vi "Text control 2 v4.7_pump-specific.vi"() -> ()   [LabVIEW 2016]
panel:
  in  "Tab Control":enum32{"Main", "Other parameters"}(tab)
  out "Line running":i32
  out "Total lines":i32
  out "Path":path=path "C:/users/rlp38/09Apr2009LTtesting/test2.txt"
  out "I vs Vg":cluster{"Y data in":dbl[], "X data in":dbl[]}[](graph)
  out "Is":dbl format="%.2e"
  out "Id":dbl format="%.2e"
  out "Ig":dbl format="%.2e"
  out "Id max vs time":cluster{"Y data in":dbl[], "X data in":dbl[]}[](graph)
  out "Id min vs time":cluster{"Y data in":dbl[], "X data in":dbl[]}[](graph)
  out "I vs Vd":cluster{"Y data in":dbl[], "X data in":dbl[]}[](graph)
  in  "Program":string="# Set time units to minutes.\n# Change filenames\n#-------------------------------------------------------\n# Port settings\n# Port 1: Nothing\n# Port 2: To sample\n# Port 3: Ultrapure water\n# Port 4: Nothing\n# Port 5: Nothing\n# Port 6: Nothing\n#-------------------------------------------------------\n# Execution time: 8 x 30 = 240 minutes = 4 hours\n# This script is designed to perform a cycling experiment between two liquids.\n# There are 8 pumping cycles, each one followed by 30 minutes of measurements.\n# All cycles pump ultrapure water (port 3).\n# Flow V = 20 pulses/second (400 ul/min)\n#-------------------------------------------------------\n# Cycle 1\npump /1ZR #initialize pump\npump /1Q #query pump\nwait-min 1 #wait 1 minute\npump /1N0R #set step resolution: 0.01 mm\npump /1Q #query pump\nwait 1000 #wait 1 second\npump /1V300R #choose speed: 300 steps/s\npump /1Q #query pump\nwait 1000 #wait 1 second\npump /1O3R #go to port 3, counterclockwise rotation\npump /1Q #query pump\nwait 1000 #wait 1 second\npump /1A2400R #go to absolute position 2400\nwait 20000 #wait 20 seconds\npump /1V20R #set speed to 20 steps/s\npump /1Q #query pump\nwait 10000 # wait 10 seconds\npump /1O2R #switch to port 2, counterclockwise rotation\npump /1Q #query pump\nwait 200 #wait 200 milliseconds\npump /1A0R #go to absolute position 0 (= empty syringe)\ntransfer d 1 -1 -0.1 -1 -1 0\npump /1Q #query pump\ntransfer d 1 -1 -0.1 -1 -1 0\npump /1? #report absolute plunger position\ntransfer d 1 -1 -0.1 -1 -1 0\nwait-min 1\npump /1Q #query pump\npump /1? #report absolute plunger position\ntransfer d 1 -1 -0.1 -1 -1 0\nwait-min 1\npump /1Q #query pump\npump /1? #report absolute plunger position\ntransfer d 1 -1 -0.1 -1 -1 0\nwait-min 1\npump /1Q #query pump\npump /1? #report absolute plunger position\ntransfer d 1 -1 -0.1 -1 -1 0\nwait-min 1\npump /1Q #query pump\npump /1? #report absolute plunger position\ntransfer d 1 -1 -0.1 -1 -1 0\nwait-min 1\npump /1Q #query pump\npump /1? #report absolute plunger position\ntransfer d 1 -1 -0.1 -1 -1 0\nwait-min 1\npump /1Q #query pump\npump /1? #report absolute plunger position\ntransfer d 1 -1 -0.1 -1 -1 0\nwait-min 1\npump /1Q #query pump\npump /1? #report absolute plunger position\ntransfer d 1 -1 -0.1 -1 -1 0\nwait-min 1\npump /1Q #query pump\npump /1? #report absolute plunger position\ntransfer d 1 -1 -0.1 -1 -1 0\nwait-min 1\npump /1Q #query pump\npump /1? #report absolute plunger position\ntransfer d 1 -1 -0.1 -1 -1 0\nwait-min 1\npump /1Q #query pump\npump /1? #report absolute plunger position\ntransfer d 1 -1 -0.1 -1 -1 0\nwait-min 1\npump /1Q #query pump\npump /1? #report absolute plunger position\ntransfer d 1 -1 -0.1 -1 -1 0\nwait-min 1\npump /1Q #query pump\npump /1? #report absolute plunger position\ntransfer d 1 -1 -0.1 -1 -1 0\nwait-min 1\npump /1Q #query pump\npump /1? #report absolute plunger position\ntransfer d 1 -1 -0.1 -1 -1 0\nwait-min 1\npump /1Q #query pump\npump /1? #report absolute plunger position\ntransfer d 1 -1 -0.1 -1 -1 0\nwait-min 1\npump /1Q #query pump\npump /1? #report absolute plunger position\ntransfer d 1 -1 -0.1 -1 -1 0\nwait-min 1\npump /1Q #query pump\npump /1? #report absolute plunger position\ntransfer d 1 -1 -0.1 -1 -1 0\nwait-min 1\npump /1Q #query pump\npump /1? #report absolute plunger position\ntransfer d 1 -1 -0.1 -1 -1 0\nwait-min 1\npump /1Q #query pump\npump /1? #report absolute plunger position\ntransfer d 1 -1 -0.1 -1 -1 0\nwait-min 1\npump /1Q #query pump\npump /1? #report absolute plunger position\ntransfer d 1 -1 -0.1 -1 -1 0\nwait-min 1\npump /1Q #query pump\npump /1? #report absolute plunger position\ntransfer d 1 -1 -0.1 -1 -1 0\nwait-min 1\npump /1Q #query pump\npump /1? #report absolute plunger position\ntransfer d 1 -1 -0.1 -1 -1 0\nwait-min 1\npump /1Q #query pump\npump /1? #report absolute plunger position\ntransfer d 1 -1 -0.1 -1 -1 0\nwait-min 1\npump /1Q #query pump\npump /1? #report absolute plunger position\ntransfer d 1 -1 -0.1 -1 -1 0\nwait-min 1\npump /1Q #query pump\npump /1? #report absolute plunger position\ntransfer d 1 -1 -0.1 -1 -1 0\nwait-min 1\n#-------------------------------------------------------\n# Cycle 2\npump /1ZR #initialize pump\npump /1Q #query pump\nwait-min 1 #wait 1 minute\npump /1N0R #set step resolution: 0.01 mm\npump /1Q #query pump\nwait 1000 #wait 1 second\npump /1V300R #choose speed: 300 steps/s\npump /1Q #query pump\nwait 1000 #wait 1 second\npump /1O3R #go to port 3, counterclockwise rotation\npump /1Q #query pump\nwait 1000 #wait 1 second\npump /1A2400R #go to absolute position 2400\nwait 30000 #wait 30 seconds \npump /1V20R #set speed to 20 steps/s\npump /1Q #query pump\nwait 10000 # wait 10 seconds\npump /1O2R #switch to port 2, counterclockwise rotation\npump /1Q #query pump\nwait 200 #wait 200 milliseconds\npump /1A0R #go to absolute position 0 (= empty syringe)\ntransfer d 1 -1 -0.1 -1 -1 0\npump /1Q #query pump\ntransfer d 1 -1 -0.1 -1 -1 0\npump /1? #report absolute plunger position\ntransfer d 1 -1 -0.1 -1 -1 0\nwait-min 1\npump /1Q #query pump\npump /1? #report absolute plunger position\ntransfer d 1 -1 -0.1 -1 -1 0\nwait-min 1\npump /1Q #query pump\npump /1? #report absolute plunger position\ntransfer d 1 -1 -0.1 -1 -1 0\nwait-min 1\npump /1Q #query pump\npump /1? #report absolute plunger position\ntransfer d 1 -1 -0.1 -1 -1 0\nwait-min 1\npump /1Q #query pump\npump /1? #report absolute plunger position\ntransfer d 1 -1 -0.1 -1 -1 0\nwait-min 1\npump /1Q #query pump\npump /1? #report absolute plunger position\ntransfer d 1 -1 -0.1 -1 -1 0\nwait-min 1\npump /1Q #query pump\npump /1? #report absolute plunger position\ntransfer d 1 -1 -0.1 -1 -1 0\nwait-min 1\npump /1Q #query pump\npump /1? #report absolute plunger position\ntransfer d 1 -1 -0.1 -1 -1 0\nwait-min 1\npump /1Q #query pump\npump /1? #report absolute plunger position\ntransfer d 1 -1 -0.1 -1 -1 0\nwait-min 1\npump /1Q #query pump\npump /1? #report absolute plunger position\ntransfer d 1 -1 -0.1 -1 -1 0\nwait-min 1\npump /1Q #query pump\npump /1? #report absolute plunger position\ntransfer d 1 -1 -0.1 -1 -1 0\nwait-min 1\npump /1Q #query pump\npump /1? #report absolute plunger position\ntransfer d 1 -1 -0.1 -1 -1 0\nwait-min 1\npump /1Q #query pump\npump /1? #report absolute plunger position\ntransfer d 1 -1 -0.1 -1 -1 0\nwait-min 1\npump /1Q #query pump\npump /1? #report absolute plunger position\ntransfer d 1 -1 -0.1 -1 -1 0\nwait-min 1\npump /1Q #query pump\npump /1? #report absolute plunger position\ntransfer d 1 -1 -0.1 -1 -1 0\nwait-min 1\npump /1Q #query pump\npump /1? #report absolute plunger position\ntransfer d 1 -1 -0.1 -1 -1 0\nwait-min 1\npump /1Q #query pump\npump /1? #report absolute plunger position\ntransfer d 1 -1 -0.1 -1 -1 0\nwait-min 1\npump /1Q #query pump\npump /1? #report absolute plunger position\ntransfer d 1 -1 -0.1 -1 -1 0\nwait-min 1\npump /1Q #query pump\npump /1? #report absolute plunger position\ntransfer d 1 -1 -0.1 -1 -1 0\nwait-min 1\npump /1Q #query pump\npump /1? #report absolute plunger position\ntransfer d 1 -1 -0.1 -1 -1 0\nwait-min 1\npump /1Q #query pump\npump /1? #report absolute plunger position\ntransfer d 1 -1 -0.1 -1 -1 0\nwait-min 1\npump /1Q #query pump\npump /1? #report absolute plunger position\ntransfer d 1 -1 -0.1 -1 -1 0\nwait-min 1\npump /1Q #query pump\npump /1? #report absolute plunger position\ntransfer d 1 -1 -0.1 -1 -1 0\nwait-min 1\npump /1Q #query pump\npump /1? #report absolute plunger position\ntransfer d 1 -1 -0.1 -1 -1 0\nwait-min 1\npump /1Q #query pump\npump /1? #report absolute plunger position\ntransfer d 1 -1 -0.1 -1 -1 0\nwait-min 1\n#-------------------------------------------------------\n# Cycle 3\npump /1ZR #initialize pump\npump /1Q #query pump\nwait-min 1 #wait 1 minute\npump /1N0R #set step resolution: 0.01 mm\npump /1Q #query pump\nwait 1000 #wait 1 second\npump /1V300R #choose speed: 300 steps/s\npump /1Q #query pump\nwait 1000 #wait 1 second\npump /1O3R #go to port 3, counterclockwise rotation\npump /1Q #query pump\nwait 1000 #wait 1 second\npump /1A2400R #go to absolute position 2400\nwait 30000 #wait 30 seconds \npump /1V20R #set speed to 20 steps/s\npump /1Q #query pump\nwait 10000 # wait 10 seconds\npump /1O2R #switch to port 2, counterclockwise rotation\npump /1Q #query pump\nwait 200 #wait 200 milliseconds\npump /1A0R #go to absolute position 0 (= empty syringe)\ntransfer d 1 -1 -0.1 -1 -1 0\npump /1Q #query pump\ntransfer d 1 -1 -0.1 -1 -1 0\npump /1? #report absolute plunger position\ntransfer d 1 -1 -0.1 -1 -1 0\nwait-min 1\npump /1Q #query pump\npump /1? #report absolute plunger position\ntransfer d 1 -1 -0.1 -1 -1 0\nwait-min 1\npump /1Q #query pump\npump /1? #report absolute plunger position\ntransfer d 1 -1 -0.1 -1 -1 0\nwait-min 1\npump /1Q #query pump\npump /1? #report absolute plunger position\ntransfer d 1 -1 -0.1 -1 -1 0\nwait-min 1\npump /1Q #query pump\npump /1? #report absolute plunger position\ntransfer d 1 -1 -0.1 -1 -1 0\nwait-min 1\npump /1Q #query pump\npump /1? #report absolute plunger position\ntransfer d 1 -1 -0.1 -1 -1 0\nwait-min 1\npump /1Q #query pump\npump /1? #report absolute plunger position\ntransfer d 1 -1 -0.1 -1 -1 0\nwait-min 1\npump /1Q #query pump\npump /1? #report absolute plunger position\ntransfer d 1 -1 -0.1 -1 -1 0\nwait-min 1\npump /1Q #query pump\npump /1? #report absolute plunger position\ntransfer d 1 -1 -0.1 -1 -1 0\nwait-min 1\npump /1Q #query pump\npump /1? #report absolute plunger position\ntransfer d 1 -1 -0.1 -1 -1 0\nwait-min 1\npump /1Q #query pump\npump /1? #report absolute plunger position\ntransfer d 1 -1 -0.1 -1 -1 0\nwait-min 1\npump /1Q #query pump\npump /1? #report absolute plunger position\ntransfer d 1 -1 -0.1 -1 -1 0\nwait-min 1\npump /1Q #query pump\npump /1? #report absolute plunger position\ntransfer d 1 -1 -0.1 -1 -1 0\nwait-min 1\npump /1Q #query pump\npump /1? #report absolute plunger position\ntransfer d 1 -1 -0.1 -1 -1 0\nwait-min 1\npump /1Q #query pump\npump /1? #report absolute plunger position\ntransfer d 1 -1 -0.1 -1 -1 0\nwait-min 1\npump /1Q #query pump\npump /1? #report absolute plunger position\ntransfer d 1 -1 -0.1 -1 -1 0\nwait-min 1\npump /1Q #query pump\npump /1? #report absolute plunger position\ntransfer d 1 -1 -0.1 -1 -1 0\nwait-min 1\npump /1Q #query pump\npump /1? #report absolute plunger position\ntransfer d 1 -1 -0.1 -1 -1 0\nwait-min 1\npump /1Q #query pump\npump /1? #report absolute plunger position\ntransfer d 1 -1 -0.1 -1 -1 0\nwait-min 1\npump /1Q #query pump\npump /1? #report absolute plunger position\ntransfer d 1 -1 -0.1 -1 -1 0\nwait-min 1\npump /1Q #query pump\npump /1? #report absolute plunger position\ntransfer d 1 -1 -0.1 -1 -1 0\nwait-min 1\npump /1Q #query pump\npump /1? #report absolute plunger position\ntransfer d 1 -1 -0.1 -1 -1 0\nwait-min 1\npump /1Q #query pump\npump /1? #report absolute plunger position\ntransfer d 1 -1 -0.1 -1 -1 0\nwait-min 1\npump /1Q #query pump\npump /1? #report absolute plunger position\ntransfer d 1 -1 -0.1 -1 -1 0\nwait-min 1\npump /1Q #query pump\npump /1? #report absolute plunger position\ntransfer d 1 -1 -0.1 -1 -1 0\nwait-min 1\n#-------------------------------------------------------\n# Cycle 4\npump /1ZR #initialize pump\npump /1Q #query pump\nwait-min 1 #wait 1 minute\npump /1N0R #set step resolution: 0.01 mm\npump /1Q #query pump\nwait 1000 #wait 1 second\npump /1V300R #choose speed: 300 steps/s\npump /1Q #query pump\nwait 1000 #wait 1 second\npump /1O3R #go to port 3, counterclockwise rotation\npump /1Q #query pump\nwait 1000 #wait 1 second\npump /1A2400R #go to absolute position 2400\nwait 30000 #wait 30 seconds \npump /1V20R #set speed to 20 steps/s\npump /1Q #query pump\nwait 10000 # wait 10 seconds\npump /1O2R #switch to port 2, counterclockwise rotation\npump /1Q #query pump\nwait 200 #wait 200 milliseconds\npump /1A0R #go to absolute position 0 (= empty syringe)\ntransfer d 1 -1 -0.1 -1 -1 0\npump /1Q #query pump\ntransfer d 1 -1 -0.1 -1 -1 0\npump /1? #report absolute plunger position\ntransfer d 1 -1 -0.1 -1 -1 0\nwait-min 1\npump /1Q #query pump\npump /1? #report absolute plunger position\ntransfer d 1 -1 -0.1 -1 -1 0\nwait-min 1\npump /1Q #query pump\npump /1? #report absolute plunger position\ntransfer d 1 -1 -0.1 -1 -1 0\nwait-min 1\npump /1Q #query pump\npump /1? #report absolute plunger position\ntransfer d 1 -1 -0.1 -1 -1 0\nwait-min 1\npump /1Q #query pump\npump /1? #report absolute plunger position\ntransfer d 1 -1 -0.1 -1 -1 0\nwait-min 1\npump /1Q #query pump\npump /1? #report absolute plunger position\ntransfer d 1 -1 -0.1 -1 -1 0\nwait-min 1\npump /1Q #query pump\npump /1? #report absolute plunger position\ntransfer d 1 -1 -0.1 -1 -1 0\nwait-min 1\npump /1Q #query pump\npump /1? #report absolute plunger position\ntransfer d 1 -1 -0.1 -1 -1 0\nwait-min 1\npump /1Q #query pump\npump /1? #report absolute plunger position\ntransfer d 1 -1 -0.1 -1 -1 0\nwait-min 1\npump /1Q #query pump\npump /1? #report absolute plunger position\ntransfer d 1 -1 -0.1 -1 -1 0\nwait-min 1\npump /1Q #query pump\npump /1? #report absolute plunger position\ntransfer d 1 -1 -0.1 -1 -1 0\nwait-min 1\npump /1Q #query pump\npump /1? #report absolute plunger position\ntransfer d 1 -1 -0.1 -1 -1 0\nwait-min 1\npump /1Q #query pump\npump /1? #report absolute plunger position\ntransfer d 1 -1 -0.1 -1 -1 0\nwait-min 1\npump /1Q #query pump\npump /1? #report absolute plunger position\ntransfer d 1 -1 -0.1 -1 -1 0\nwait-min 1\npump /1Q #query pump\npump /1? #report absolute plunger position\ntransfer d 1 -1 -0.1 -1 -1 0\nwait-min 1\npump /1Q #query pump\npump /1? #report absolute plunger position\ntransfer d 1 -1 -0.1 -1 -1 0\nwait-min 1\npump /1Q #query pump\npump /1? #report absolute plunger position\ntransfer d 1 -1 -0.1 -1 -1 0\nwait-min 1\npump /1Q #query pump\npump /1? #report absolute plunger position\ntransfer d 1 -1 -0.1 -1 -1 0\nwait-min 1\npump /1Q #query pump\npump /1? #report absolute plunger position\ntransfer d 1 -1 -0.1 -1 -1 0\nwait-min 1\npump /1Q #query pump\npump /1? #report absolute plunger position\ntransfer d 1 -1 -0.1 -1 -1 0\nwait-min 1\npump /1Q #query pump\npump /1? #report absolute plunger position\ntransfer d 1 -1 -0.1 -1 -1 0\nwait-min 1\npump /1Q #query pump\npump /1? #report absolute plunger position\ntransfer d 1 -1 -0.1 -1 -1 0\nwait-min 1\npump /1Q #query pump\npump /1? #report absolute plunger position\ntransfer d 1 -1 -0.1 -1 -1 0\nwait-min 1\npump /1Q #query pump\npump /1? #report absolute plunger position\ntransfer d 1 -1 -0.1 -1 -1 0\nwait-min 1\npump /1Q #query pump\npump /1? #report absolute plunger position\ntransfer d 1 -1 -0.1 -1 -1 0\nwait-min 1\n#-------------------------------------------------------\n# Cycle 5\npump /1ZR #initialize pump\npump /1Q #query pump\nwait-min 1 #wait 1 minute\npump /1N0R #set step resolution: 0.01 mm\npump /1Q #query pump\nwait 1000 #wait 1 second\npump /1V300R #choose speed: 300 steps/s\npump /1Q #query pump\nwait 1000 #wait 1 second\npump /1O3R #go to port 3, counterclockwise rotation\npump /1Q #query pump\nwait 1000 #wait 1 second\npump /1A2400R #go to absolute position 2400\nwait 20000 #wait 20 seconds\npump /1V20R #set speed to 20 steps/s\npump /1Q #query pump\nwait 10000 # wait 10 seconds\npump /1O2R #switch to port 2, counterclockwise rotation\npump /1Q #query pump\nwait 200 #wait 200 milliseconds\npump /1A0R #go to absolute position 0 (= empty syringe)\ntransfer d 1 -1 -0.1 -1 -1 0\npump /1Q #query pump\ntransfer d 1 -1 -0.1 -1 -1 0\npump /1? #report absolute plunger position\ntransfer d 1 -1 -0.1 -1 -1 0\nwait-min 1\npump /1Q #query pump\npump /1? #report absolute plunger position\ntransfer d 1 -1 -0.1 -1 -1 0\nwait-min 1\npump /1Q #query pump\npump /1? #report absolute plunger position\ntransfer d 1 -1 -0.1 -1 -1 0\nwait-min 1\npump /1Q #query pump\npump /1? #report absolute plunger position\ntransfer d 1 -1 -0.1 -1 -1 0\nwait-min 1\npump /1Q #query pump\npump /1? #report absolute plunger position\ntransfer d 1 -1 -0.1 -1 -1 0\nwait-min 1\npump /1Q #query pump\npump /1? #report absolute plunger position\ntransfer d 1 -1 -0.1 -1 -1 0\nwait-min 1\npump /1Q #query pump\npump /1? #report absolute plunger position\ntransfer d 1 -1 -0.1 -1 -1 0\nwait-min 1\npump /1Q #query pump\npump /1? #report absolute plunger position\ntransfer d 1 -1 -0.1 -1 -1 0\nwait-min 1\npump /1Q #query pump\npump /1? #report absolute plunger position\ntransfer d 1 -1 -0.1 -1 -1 0\nwait-min 1\npump /1Q #query pump\npump /1? #report absolute plunger position\ntransfer d 1 -1 -0.1 -1 -1 0\nwait-min 1\npump /1Q #query pump\npump /1? #report absolute plunger position\ntransfer d 1 -1 -0.1 -1 -1 0\nwait-min 1\npump /1Q #query pump\npump /1? #report absolute plunger position\ntransfer d 1 -1 -0.1 -1 -1 0\nwait-min 1\npump /1Q #query pump\npump /1? #report absolute plunger position\ntransfer d 1 -1 -0.1 -1 -1 0\nwait-min 1\npump /1Q #query pump\npump /1? #report absolute plunger position\ntransfer d 1 -1 -0.1 -1 -1 0\nwait-min 1\npump /1Q #query pump\npump /1? #report absolute plunger position\ntransfer d 1 -1 -0.1 -1 -1 0\nwait-min 1\npump /1Q #query pump\npump /1? #report absolute plunger position\ntransfer d 1 -1 -0.1 -1 -1 0\nwait-min 1\npump /1Q #query pump\npump /1? #report absolute plunger position\ntransfer d 1 -1 -0.1 -1 -1 0\nwait-min 1\npump /1Q #query pump\npump /1? #report absolute plunger position\ntransfer d 1 -1 -0.1 -1 -1 0\nwait-min 1\npump /1Q #query pump\npump /1? #report absolute plunger position\ntransfer d 1 -1 -0.1 -1 -1 0\nwait-min 1\npump /1Q #query pump\npump /1? #report absolute plunger position\ntransfer d 1 -1 -0.1 -1 -1 0\nwait-min 1\npump /1Q #query pump\npump /1? #report absolute plunger position\ntransfer d 1 -1 -0.1 -1 -1 0\nwait-min 1\npump /1Q #query pump\npump /1? #report absolute plunger position\ntransfer d 1 -1 -0.1 -1 -1 0\nwait-min 1\npump /1Q #query pump\npump /1? #report absolute plunger position\ntransfer d 1 -1 -0.1 -1 -1 0\nwait-min 1\npump /1Q #query pump\npump /1? #report absolute plunger position\ntransfer d 1 -1 -0.1 -1 -1 0\nwait-min 1\npump /1Q #query pump\npump /1? #report absolute plunger position\ntransfer d 1 -1 -0.1 -1 -1 0\nwait-min 1\n#-------------------------------------------------------\n# Cycle 6\npump /1ZR #initialize pump\npump /1Q #query pump\nwait-min 1 #wait 1 minute\npump /1N0R #set step resolution: 0.01 mm\npump /1Q #query pump\nwait 1000 #wait 1 second\npump /1V300R #choose speed: 300 steps/s\npump /1Q #query pump\nwait 1000 #wait 1 second\npump /1O3R #go to port 3, counterclockwise rotation\npump /1Q #query pump\nwait 1000 #wait 1 second\npump /1A2400R #go to absolute position 2400\nwait 30000 #wait 30 seconds \npump /1V20R #set speed to 20 steps/s\npump /1Q #query pump\nwait 10000 # wait 10 seconds\npump /1O2R #switch to port 2, counterclockwise rotation\npump /1Q #query pump\nwait 200 #wait 200 milliseconds\npump /1A0R #go to absolute position 0 (= empty syringe)\ntransfer d 1 -1 -0.1 -1 -1 0\npump /1Q #query pump\ntransfer d 1 -1 -0.1 -1 -1 0\npump /1? #report absolute plunger position\ntransfer d 1 -1 -0.1 -1 -1 0\nwait-min 1\npump /1Q #query pump\npump /1? #report absolute plunger position\ntransfer d 1 -1 -0.1 -1 -1 0\nwait-min 1\npump /1Q #query pump\npump /1? #report absolute plunger position\ntransfer d 1 -1 -0.1 -1 -1 0\nwait-min 1\npump /1Q #query pump\npump /1? #report absolute plunger position\ntransfer d 1 -1 -0.1 -1 -1 0\nwait-min 1\npump /1Q #query pump\npump /1? #report absolute plunger position\ntransfer d 1 -1 -0.1 -1 -1 0\nwait-min 1\npump /1Q #query pump\npump /1? #report absolute plunger position\ntransfer d 1 -1 -0.1 -1 -1 0\nwait-min 1\npump /1Q #query pump\npump /1? #report absolute plunger position\ntransfer d 1 -1 -0.1 -1 -1 0\nwait-min 1\npump /1Q #query pump\npump /1? #report absolute plunger position\ntransfer d 1 -1 -0.1 -1 -1 0\nwait-min 1\npump /1Q #query pump\npump /1? #report absolute plunger position\ntransfer d 1 -1 -0.1 -1 -1 0\nwait-min 1\npump /1Q #query pump\npump /1? #report absolute plunger position\ntransfer d 1 -1 -0.1 -1 -1 0\nwait-min 1\npump /1Q #query pump\npump /1? #report absolute plunger position\ntransfer d 1 -1 -0.1 -1 -1 0\nwait-min 1\npump /1Q #query pump\npump /1? #report absolute plunger position\ntransfer d 1 -1 -0.1 -1 -1 0\nwait-min 1\npump /1Q #query pump\npump /1? #report absolute plunger position\ntransfer d 1 -1 -0.1 -1 -1 0\nwait-min 1\npump /1Q #query pump\npump /1? #report absolute plunger position\ntransfer d 1 -1 -0.1 -1 -1 0\nwait-min 1\npump /1Q #query pump\npump /1? #report absolute plunger position\ntransfer d 1 -1 -0.1 -1 -1 0\nwait-min 1\npump /1Q #query pump\npump /1? #report absolute plunger position\ntransfer d 1 -1 -0.1 -1 -1 0\nwait-min 1\npump /1Q #query pump\npump /1? #report absolute plunger position\ntransfer d 1 -1 -0.1 -1 -1 0\nwait-min 1\npump /1Q #query pump\npump /1? #report absolute plunger position\ntransfer d 1 -1 -0.1 -1 -1 0\nwait-min 1\npump /1Q #query pump\npump /1? #report absolute plunger position\ntransfer d 1 -1 -0.1 -1 -1 0\nwait-min 1\npump /1Q #query pump\npump /1? #report absolute plunger position\ntransfer d 1 -1 -0.1 -1 -1 0\nwait-min 1\npump /1Q #query pump\npump /1? #report absolute plunger position\ntransfer d 1 -1 -0.1 -1 -1 0\nwait-min 1\npump /1Q #query pump\npump /1? #report absolute plunger position\ntransfer d 1 -1 -0.1 -1 -1 0\nwait-min 1\npump /1Q #query pump\npump /1? #report absolute plunger position\ntransfer d 1 -1 -0.1 -1 -1 0\nwait-min 1\npump /1Q #query pump\npump /1? #report absolute plunger position\ntransfer d 1 -1 -0.1 -1 -1 0\nwait-min 1\npump /1Q #query pump\npump /1? #report absolute plunger position\ntransfer d 1 -1 -0.1 -1 -1 0\nwait-min 1\n#-------------------------------------------------------\n# Cycle 7\npump /1ZR #initialize pump\npump /1Q #query pump\nwait-min 1 #wait 1 minute\npump /1N0R #set step resolution: 0.01 mm\npump /1Q #query pump\nwait 1000 #wait 1 second\npump /1V300R #choose speed: 300 steps/s\npump /1Q #query pump\nwait 1000 #wait 1 second\npump /1O3R #go to port 3, counterclockwise rotation\npump /1Q #query pump\nwait 1000 #wait 1 second\npump /1A2400R #go to absolute position 2400\nwait 30000 #wait 30 seconds \npump /1V20R #set speed to 20 steps/s\npump /1Q #query pump\nwait 10000 # wait 10 seconds\npump /1O2R #switch to port 2, counterclockwise rotation\npump /1Q #query pump\nwait 200 #wait 200 milliseconds\npump /1A0R #go to absolute position 0 (= empty syringe)\ntransfer d 1 -1 -0.1 -1 -1 0\npump /1Q #query pump\ntransfer d 1 -1 -0.1 -1 -1 0\npump /1? #report absolute plunger position\ntransfer d 1 -1 -0.1 -1 -1 0\nwait-min 1\npump /1Q #query pump\npump /1? #report absolute plunger position\ntransfer d 1 -1 -0.1 -1 -1 0\nwait-min 1\npump /1Q #query pump\npump /1? #report absolute plunger position\ntransfer d 1 -1 -0.1 -1 -1 0\nwait-min 1\npump /1Q #query pump\npump /1? #report absolute plunger position\ntransfer d 1 -1 -0.1 -1 -1 0\nwait-min 1\npump /1Q #query pump\npump /1? #report absolute plunger position\ntransfer d 1 -1 -0.1 -1 -1 0\nwait-min 1\npump /1Q #query pump\npump /1? #report absolute plunger position\ntransfer d 1 -1 -0.1 -1 -1 0\nwait-min 1\npump /1Q #query pump\npump /1? #report absolute plunger position\ntransfer d 1 -1 -0.1 -1 -1 0\nwait-min 1\npump /1Q #query pump\npump /1? #report absolute plunger position\ntransfer d 1 -1 -0.1 -1 -1 0\nwait-min 1\npump /1Q #query pump\npump /1? #report absolute plunger position\ntransfer d 1 -1 -0.1 -1 -1 0\nwait-min 1\npump /1Q #query pump\npump /1? #report absolute plunger position\ntransfer d 1 -1 -0.1 -1 -1 0\nwait-min 1\npump /1Q #query pump\npump /1? #report absolute plunger position\ntransfer d 1 -1 -0.1 -1 -1 0\nwait-min 1\npump /1Q #query pump\npump /1? #report absolute plunger position\ntransfer d 1 -1 -0.1 -1 -1 0\nwait-min 1\npump /1Q #query pump\npump /1? #report absolute plunger position\ntransfer d 1 -1 -0.1 -1 -1 0\nwait-min 1\npump /1Q #query pump\npump /1? #report absolute plunger position\ntransfer d 1 -1 -0.1 -1 -1 0\nwait-min 1\npump /1Q #query pump\npump /1? #report absolute plunger position\ntransfer d 1 -1 -0.1 -1 -1 0\nwait-min 1\npump /1Q #query pump\npump /1? #report absolute plunger position\ntransfer d 1 -1 -0.1 -1 -1 0\nwait-min 1\npump /1Q #query pump\npump /1? #report absolute plunger position\ntransfer d 1 -1 -0.1 -1 -1 0\nwait-min 1\npump /1Q #query pump\npump /1? #report absolute plunger position\ntransfer d 1 -1 -0.1 -1 -1 0\nwait-min 1\npump /1Q #query pump\npump /1? #report absolute plunger position\ntransfer d 1 -1 -0.1 -1 -1 0\nwait-min 1\npump /1Q #query pump\npump /1? #report absolute plunger position\ntransfer d 1 -1 -0.1 -1 -1 0\nwait-min 1\npump /1Q #query pump\npump /1? #report absolute plunger position\ntransfer d 1 -1 -0.1 -1 -1 0\nwait-min 1\npump /1Q #query pump\npump /1? #report absolute plunger position\ntransfer d 1 -1 -0.1 -1 -1 0\nwait-min 1\npump /1Q #query pump\npump /1? #report absolute plunger position\ntransfer d 1 -1 -0.1 -1 -1 0\nwait-min 1\npump /1Q #query pump\npump /1? #report absolute plunger position\ntransfer d 1 -1 -0.1 -1 -1 0\nwait-min 1\npump /1Q #query pump\npump /1? #report absolute plunger position\ntransfer d 1 -1 -0.1 -1 -1 0\nwait-min 1\n#-------------------------------------------------------\n# Cycle 8\npump /1ZR #initialize pump\npump /1Q #query pump\nwait-min 1 #wait 1 minute\npump /1N0R #set step resolution: 0.01 mm\npump /1Q #query pump\nwait 1000 #wait 1 second\npump /1V300R #choose speed: 300 steps/s\npump /1Q #query pump\nwait 1000 #wait 1 second\npump /1O3R #go to port 3, counterclockwise rotation\npump /1Q #query pump\nwait 1000 #wait 1 second\npump /1A2400R #go to absolute position 2400\nwait 30000 #wait 30 seconds \npump /1V20R #set speed to 20 steps/s\npump /1Q #query pump\nwait 10000 # wait 10 seconds\npump /1O2R #switch to port 2, counterclockwise rotation\npump /1Q #query pump\nwait 200 #wait 200 milliseconds\npump /1A0R #go to absolute position 0 (= empty syringe)\ntransfer d 1 -1 -0.1 -1 -1 0\npump /1Q #query pump\ntransfer d 1 -1 -0.1 -1 -1 0\npump /1? #report absolute plunger position\ntransfer d 1 -1 -0.1 -1 -1 0\nwait-min 1\npump /1Q #query pump\npump /1? #report absolute plunger position\ntransfer d 1 -1 -0.1 -1 -1 0\nwait-min 1\npump /1Q #query pump\npump /1? #report absolute plunger position\ntransfer d 1 -1 -0.1 -1 -1 0\nwait-min 1\npump /1Q #query pump\npump /1? #report absolute plunger position\ntransfer d 1 -1 -0.1 -1 -1 0\nwait-min 1\npump /1Q #query pump\npump /1? #report absolute plunger position\ntransfer d 1 -1 -0.1 -1 -1 0\nwait-min 1\npump /1Q #query pump\npump /1? #report absolute plunger position\ntransfer d 1 -1 -0.1 -1 -1 0\nwait-min 1\npump /1Q #query pump\npump /1? #report absolute plunger position\ntransfer d 1 -1 -0.1 -1 -1 0\nwait-min 1\npump /1Q #query pump\npump /1? #report absolute plunger position\ntransfer d 1 -1 -0.1 -1 -1 0\nwait-min 1\npump /1Q #query pump\npump /1? #report absolute plunger position\ntransfer d 1 -1 -0.1 -1 -1 0\nwait-min 1\npump /1Q #query pump\npump /1? #report absolute plunger position\ntransfer d 1 -1 -0.1 -1 -1 0\nwait-min 1\npump /1Q #query pump\npump /1? #report absolute plunger position\ntransfer d 1 -1 -0.1 -1 -1 0\nwait-min 1\npump /1Q #query pump\npump /1? #report absolute plunger position\ntransfer d 1 -1 -0.1 -1 -1 0\nwait-min 1\npump /1Q #query pump\npump /1? #report absolute plunger position\ntransfer d 1 -1 -0.1 -1 -1 0\nwait-min 1\npump /1Q #query pump\npump /1? #report absolute plunger position\ntransfer d 1 -1 -0.1 -1 -1 0\nwait-min 1\npump /1Q #query pump\npump /1? #report absolute plunger position\ntransfer d 1 -1 -0.1 -1 -1 0\nwait-min 1\npump /1Q #query pump\npump /1? #report absolute plunger position\ntransfer d 1 -1 -0.1 -1 -1 0\nwait-min 1\npump /1Q #query pump\npump /1? #report absolute plunger position\ntransfer d 1 -1 -0.1 -1 -1 0\nwait-min 1\npump /1Q #query pump\npump /1? #report absolute plunger position\ntransfer d 1 -1 -0.1 -1 -1 0\nwait-min 1\npump /1Q #query pump\npump /1? #report absolute plunger position\ntransfer d 1 -1 -0.1 -1 -1 0\nwait-min 1\npump /1Q #query pump\npump /1? #report absolute plunger position\ntransfer d 1 -1 -0.1 -1 -1 0\nwait-min 1\npump /1Q #query pump\npump /1? #report absolute plunger position\ntransfer d 1 -1 -0.1 -1 -1 0\nwait-min 1\npump /1Q #query pump\npump /1? #report absolute plunger position\ntransfer d 1 -1 -0.1 -1 -1 0\nwait-min 1\npump /1Q #query pump\npump /1? #report absolute plunger position\ntransfer d 1 -1 -0.1 -1 -1 0\nwait-min 1\npump /1Q #query pump\npump /1? #report absolute plunger position\ntransfer d 1 -1 -0.1 -1 -1 0\nwait-min 1\npump /1Q #query pump\npump /1? #report absolute plunger position\ntransfer d 1 -1 -0.1 -1 -1 0\nwait-min 1"
  out "Command running:":string="#output s 0 0 0 -0.008 0.008 0.002"
  out "Serial port data":string
  out "Elapsed Time":dbl caption="Elapsed Time (s)"
  in  "Units":u16(ring)=1 items=["Seconds", "Minutes", "Hours"]
  in  "Time Offset":dbl caption="Set Start Time (s)"
  in  "Reset":bool
  in  "Auto Reset":bool
  in  "integration time":u32(slide) max=2 step=1 scale=0.0..2.0
  in  "Interrupt run":bool
  out "Absolute plunger position vs time":cluster{"Y data in":dbl[], "X data in":dbl[]}[](graph)
  out "Valve position vs time":cluster{"Y data in":dbl[], "X data in":dbl[]}[](graph)
  in  "Halt pump":bool
  in  "Hard stop pump":bool
  in  "Gate Range\nmode":u16(ring) items=["Auto", "Limited", "Fixed"]
  in  "Gate Range":u8(slide)=6 max=11 scale=0.0..11.0
  in  "Source/Drain\nRange mode":u16(ring) items=["Auto", "Limited", "Fixed"]
  in  "Source/Drain Range":u8(slide)=6 max=11 scale=0.0..11.0
  in  "Panel Controls":T1={"Emergency Stop"=refnum, "TransGraph Max"=1e-05, "Text/Graph (text=false)"=TRUE} {"TransGraph Max" format="%.2e"}
  in  "Panel Controls 2":T2={"Emergency Stop"=refnum, "TransGraph Max"=1e-05, "Text/Graph (text=false)"=TRUE, "TransGraph Min"=1e-11} {"TransGraph Min" format="%.2e"; "TransGraph Max" format="%.2e"}
  in  "SMU4":cluster{"on/off":bool, "Voltage":dbl} {"Voltage" min=-100.0 max=100.0 format="%.2f"}
  in  "Full Reset":bool
  in  "Standby":T3
  out "error out":errorcluster
  in  "Delay before read (ms)":u32=1000
  in  "byte count":u32=64
  in  "Serial End Mode for Reads":u16(ring)=2 items=["None", "LastBit", "TermChar"]
  in  "Timeout (ms)":u32=10000
  in  "Enable Termination\nChar (T)":bool=TRUE
  in  "Termination char\n(0xA = '\\n' = LF)\n(0xD = '\\r' = CR)":u8=13 format="%.0x"
  in  "flow control":u16(ring) items=["None"=0, "XON/XOFF"=1, "RTS/CTS"=2, "DTR/DSR"=4]
  in  "stop bits":u16(ring)=10 items=["1.0"=10, "1.5"=15, "2.0"=20]
  in  "parity":u16(ring) items=["None", "Odd", "Even", "Mark", "Space"]
  in  "data bits":u16=8 min=5 max=8 step=1
  in  "VISA resource name":refnum<visa-resource-name>="COM6"
  in  "baud rate":u32=9600
  in  "Drain: Compliance":dbl=0.001 format="%.8f"
  in  "Gate: Compliance":dbl=0.001 format="%.8f"
  in  "hold time /s":dbl format="%.2f"
  in  "delay time /s":dbl format="%.2f"
  in  "Integration time (short)":dbl=0.0019 min=8e-05 max=0.0019 step=8e-05 format="%^.0e"
  in  "Integration time (long)":dbl=0.32 min=0.04 max=2.0 step=0.02 format="%.2f"
  in  "Step delay /s":dbl format="%.2f"
  in  "Prefix (transfer)":string="_step_1_ultrapure_H2O_"
  in  "Suffix (transfer)":string="_T.txt"
  in  "Prefix (Idmax-Idmin)":string="_step_1_ultrapure_H2O_Idmax_Idmin_vs_time_Vg=-1.0V_Vd=-1.0V"
  in  "Suffix (Idmax-Idmin)":string=".txt"
  in  "Prefix (output)":string="_step_1_ultrapure_H2O_"
  in  "Suffix (output)":string="_O.txt"
  in  "Prefix (script)":string="_step_1_ultrapure_H2O_script"
  in  "Prefix (serial port output)":string="_step_1_ultrapure_H2O_serial port output"
  in  "Prefix (plunger)":string="_step_1_ultrapure_H2O_plunger_vs_time"
  in  "Suffix (plunger)":string=".txt"
  in  "Gate":T4={"Gate Start"=0.0, "Gate Stop"=2.0, "Gate Step (linear only)"=1.0, "Gate Compliance"=0.0001, "Gate PComp"=0.0, "Range mode"=0, "Range"=6} {"Range" max=11 scale=0.0..11.0; "Range mode" items=["Auto", "Limited", "Fixed"]; "Gate PComp" format="%^.2e"; "Gate Compliance" format="%^.2e"; "Gate Step (linear only)" format="%^.4e"; "Gate Stop" format="%^.4e"; "Gate Start" format="%^.4e"}
  in  "Drain 2":T5={"Drain Start"=0.0, "Drain Stop"=2.0, "Drain Compliance"=0.0001, "Drain Step"=1.0, "Drain PComp"=0.0, "Range mode"=0, "Range"=6} {"Range" max=11 scale=0.0..11.0; "Range mode" items=["Auto", "Limited", "Fixed"]; "Drain PComp" format="%^.2e"; "Drain Step" format="%^.4e"; "Drain Compliance" format="%^.2e"; "Drain Stop" format="%^.4e"; "Drain Start" format="%^.4e"}
  in  "Timings 2":T6={"integration time"=0, "Short/Long integration time"=0.00064, "hold time (sec)"=0.0, "delay time (sec)"=0.0, "Step Time (0 disables)"=0.0, "sweep method"=0, "Pulse period"=0.005, "Base voltage"=0.0, "Pulse width"=0.0005} {"Pulse width" min=0.0005 max=0.1 step=0.0001 format="%.4f"; "Base voltage" format="%^.4e"; "Pulse period" min=0.005 max=1.0 step=0.0001 format="%.4f"; "sweep method" items=["Continuous", "Pulsed"]; "Step Time (0 disables)" format="%.2f"; "delay time (sec)" format="%.4f"; "hold time (sec)" format="%.4f"; "Short/Long integration time" format="%^.0e"; "integration time" scale=0.0..2.0}
  # "Syntax:\nitime [s|m|l]\ngaterangemode [a|l|f]\ndrainrangemode [a|l|f]\npulsed [on|off] PulsePeriod(sec) PulseBaseVoltage PulseONWidth(sec)\nstandby [on l off]\nwait NumMilliseconds\nwait-min NumMinutes\n# texthere = comment\ntransfer [s|d] VgStart VgStop VgStep VdStart VdStop VdStep\noutput [s|d] VgStart VgStop VgStep VdStart VdStop VdStep\nsample Vg Vd NumSamples Time(s) SampleInterval(s)\nsamplei Idg NumSamples Time(s) SampleInterval(s) VDGcompliance\n100 samples is approximately 13 seconds with medium integration\n# if in doubt use SampleInterval(s) = 0.004\nstressV VG VD IGcompliance IDcompliance Duration(sec)\nstressI IDG VDGcompliance Duration(sec)\nvsu2pulse Bias Duration(s)\npulsedstressV [s|d] VEstop VgON VgOFF Period(s) PulseONwidth(s) Vd\nsample-fpp Vg Vd NumSamples Time\nresample-fpp Vg Vd\ntransfer-fpp [s|d] VgStart VgStop VgStep VdStart VdStop VdStep\noutput-fpp [s|d] VgStart VgStop VgStep VdStart VdStop VdStep\nserial SerialPortCommand\npump SerialPortCommand for the OEM pump\n\nSPM OEM Pump Syntax (<x>: pump number, use 1 if only one pump):\nif the command syntax contains [R], then append the letter R to the command\n/<x>Q: query (a query command should follow each command)\n/<x>Z[R] or /<x>Y[R]: initialize pump\n/<x>N<n>[R] (<n>=0,1): <0> (<1>) microstep 0.01 mm (0.00125 mm) resolution\n/<x>I<n> (<n>=0-6): turn to port number n (clockwise)\n/<x>O<n> (<n>=0-6): turn to port number n (counterclockwise)\n/<x>X: Re-execute last command string\n/<x>G<n>[R] (<n>=0-60000): repeat command sequence (default: 0, 0=loop forever)\n/<x>g: Mark the start of a repeat sequence (max = 10)\n/<x>M<n>[R] (<n>=0-86400000): delay command execution by n milliseconds\n/<x>H: Halt; Pause the sequence after finishing the current move\n/<x>T: Hardstop; Interrupt the current move and suppress it from the sequence\n/<x>A<n>[R] (<n>=0-3000 with N=0, 0-24000 with N=1): absolute position\n/<x>P<n>[R] (<n>=0-3000 with N=0, 0-24000 with N=1): relative pickup\n/<x>D<n>[R] (<n>=0-3000 with N=0, 0-24000 with N=1): relative dispense\n/<x>V<n>[R] (<n>=5-1600 default: 150): set peak speed (pulses/sec)\n/<x>S<n>[R] (<n>=10-40 default: 22): set speed (NOT in pulses/sec, look in manual)\nNOTE: When controlled with absolute position, one does not need to pay special attention to the syringe that is mounted on the pump.\nWithdraw from lower stage (ports 3, 5), dispense from higher stage (ports 2, 4, 6).\nConnect Port 1 to waste."
  # "Time"
  # "1\n2\n3\n4\n5\n6\n7\n8\n9\n10\n11\n12\n13\n14\n15\n16\n17\n18\n19\n20"
  # "Serial port settings"
  # "Filename settings"
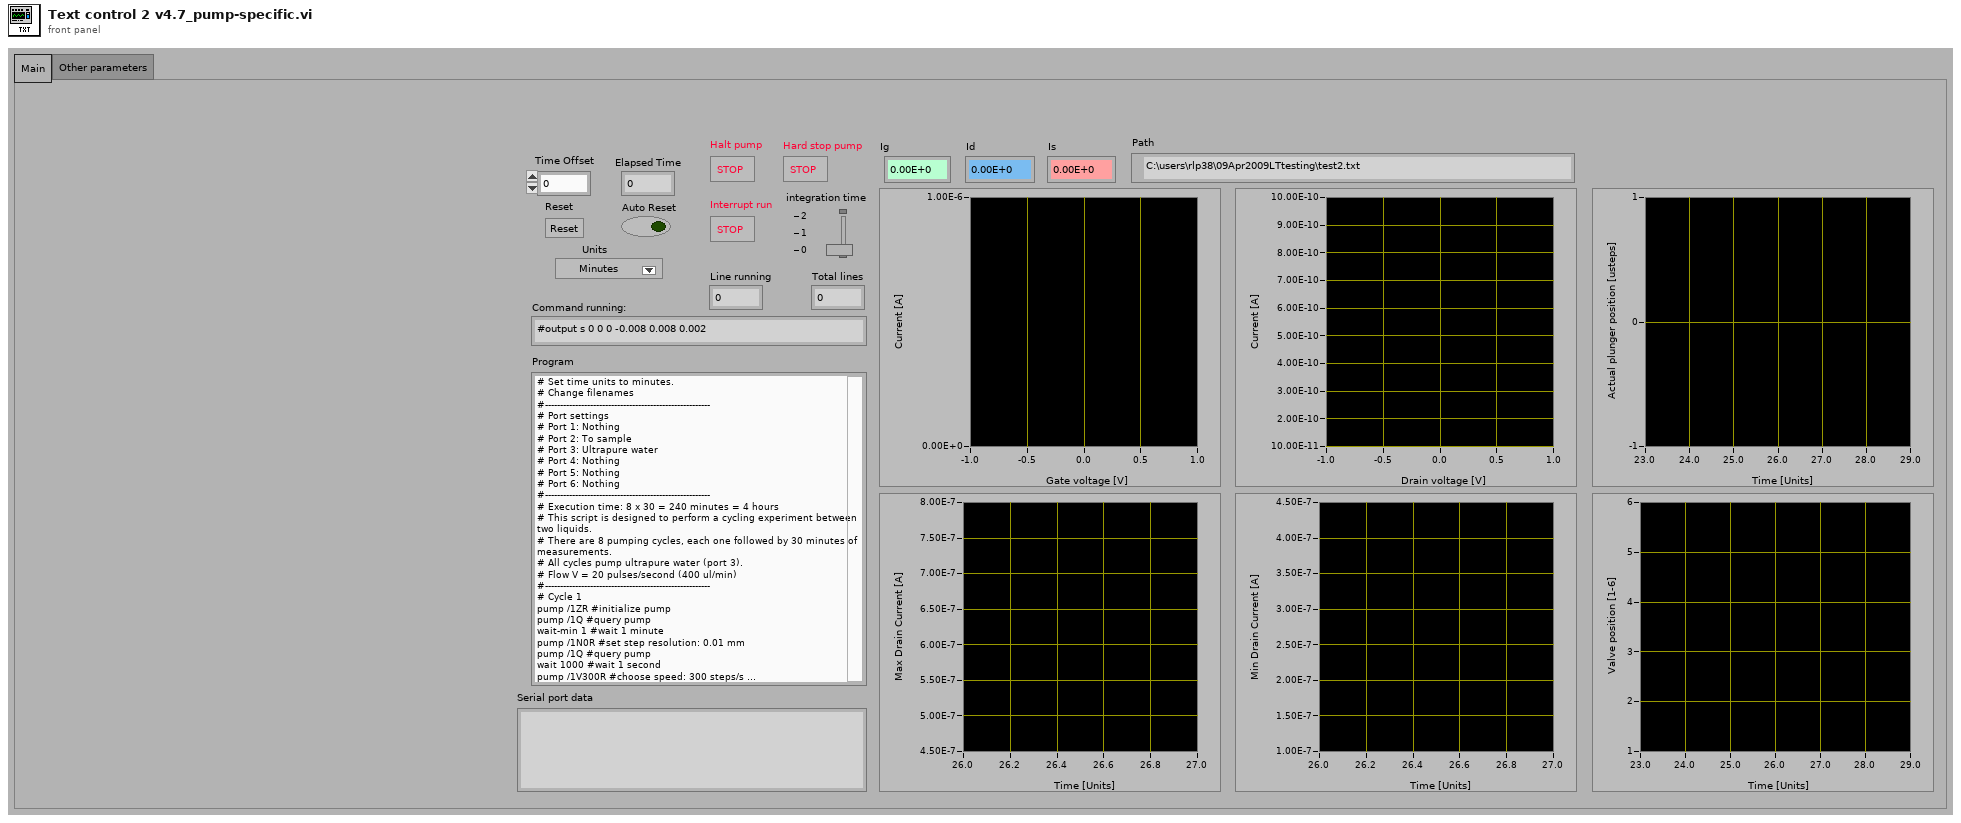
[diagram p1: front panel]
types:
  T1 = cluster{"Emergency Stop":refnum<vi>, "TransGraph Max":dbl, "Text/Graph (text=false)":bool}
  T2 = cluster{"Emergency Stop":refnum<vi>, "TransGraph Max":dbl, "Text/Graph (text=false)":bool, "TransGraph Min":dbl}
  T3 = cluster{"Gate Standby":bool, "Drain Standby":bool}
  T4 = cluster{"Gate Start":dbl, "Gate Stop":dbl, "Gate Step (linear only)":dbl, "Gate Compliance":dbl, "Gate PComp":dbl, "Range mode":u16, "Range":u8}
  T5 = cluster{"Drain Start":dbl, "Drain Stop":dbl, "Drain Compliance":dbl, "Drain Step":dbl, "Drain PComp":dbl, "Range mode":u16, "Range":u8}
  T6 = cluster{"integration time":u32, "Short/Long integration time":dbl, "hold time (sec)":dbl, "delay time (sec)":dbl, "Step Time (0 disables)":dbl, "sweep method":u16, "Pulse period":dbl, "Base voltage":dbl, "Pulse width":dbl}
  T7 = enum16{"open", "replace", "create", "open or create", "replace or create", "replace or create with confirmation"}
  T8 = cluster{"V2 Start":dbl, "V2 Step":dbl, "Number of points":i32}
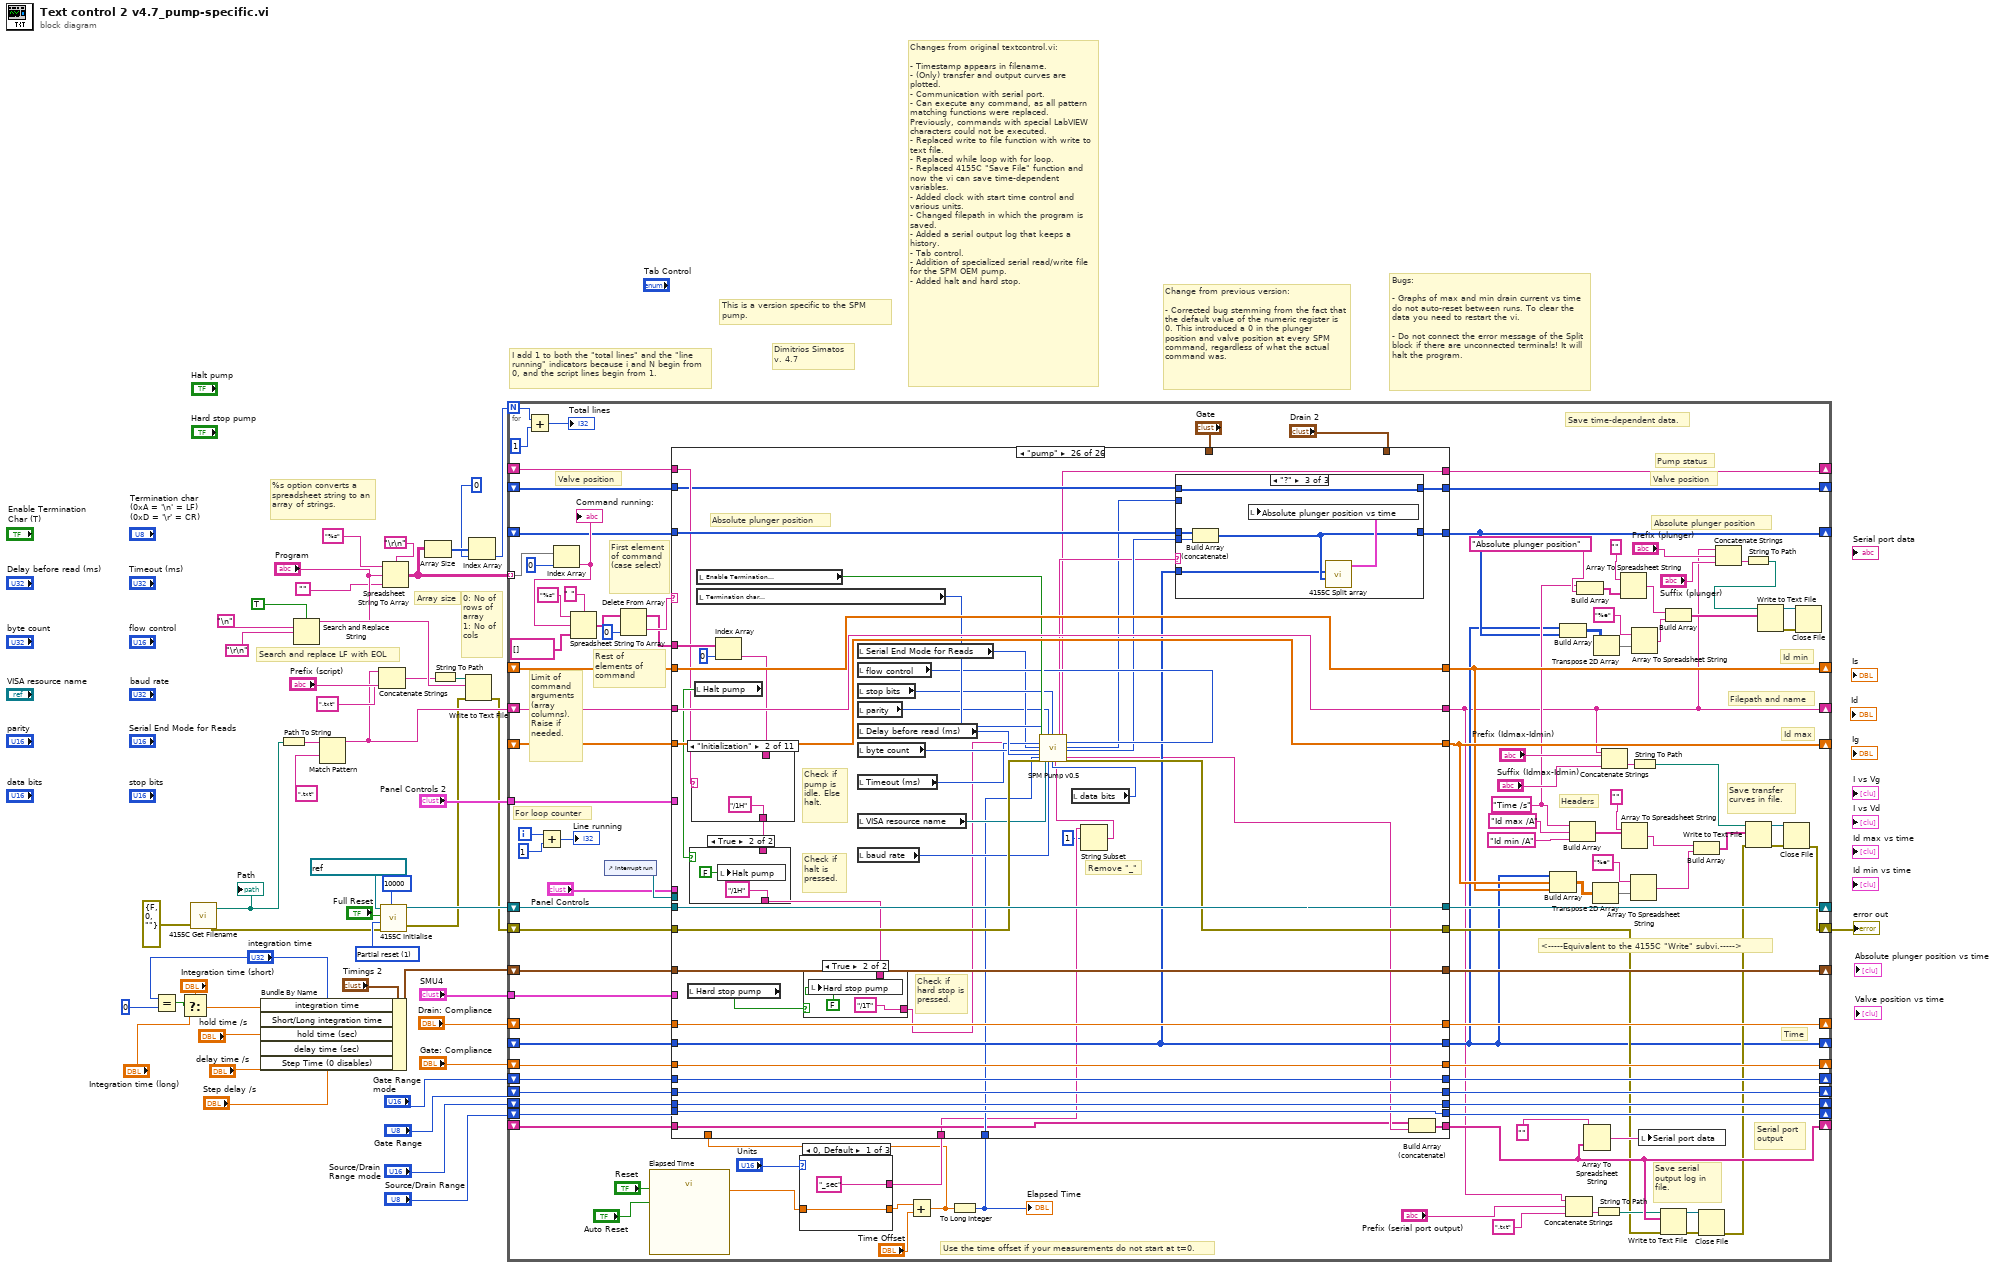
[diagram p0: block diagram]
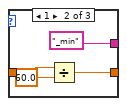
[diagram p2: hidden frame]
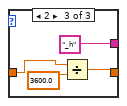
[diagram p3: hidden frame]
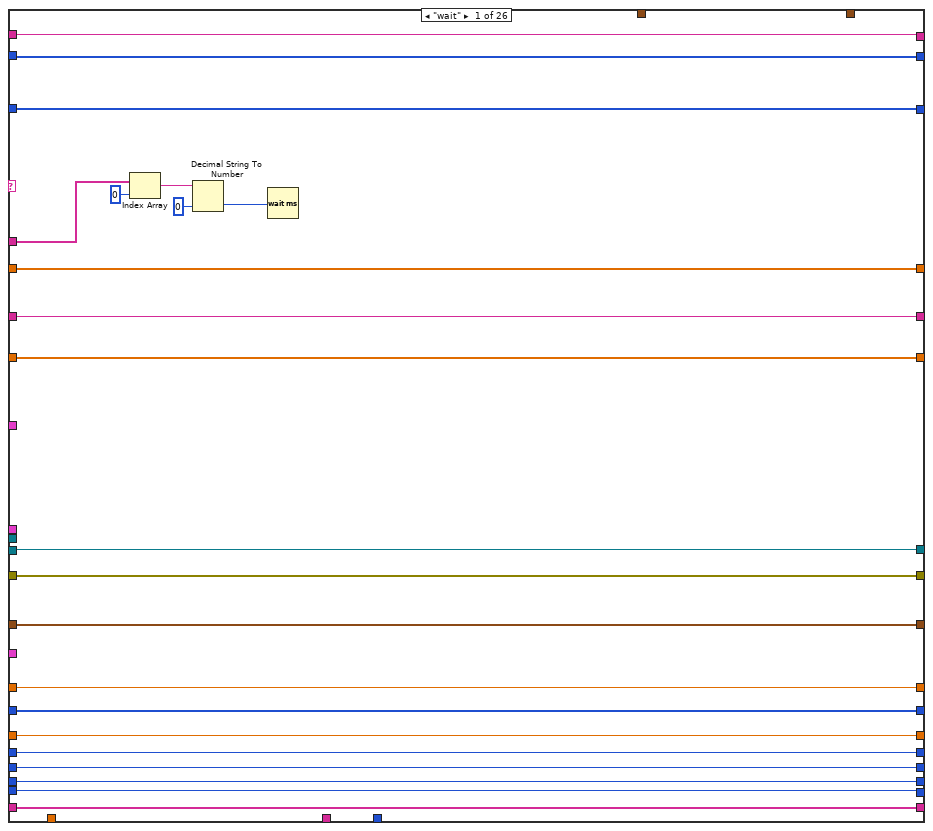
[diagram p4: hidden frame]
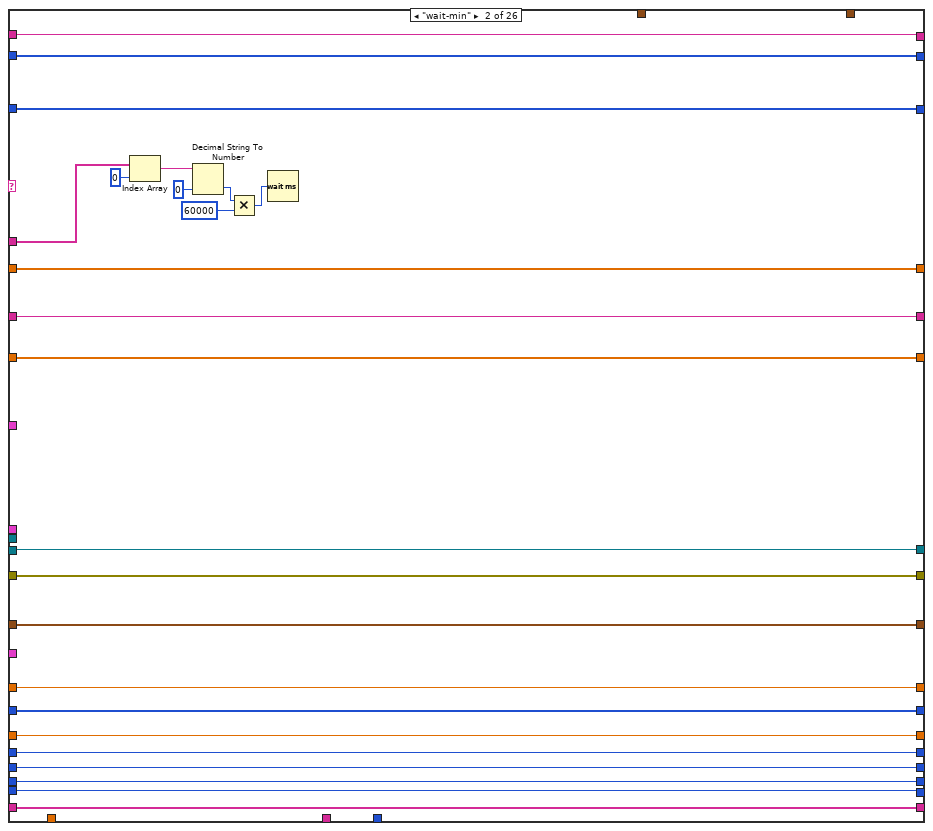
[diagram p5: hidden frame]
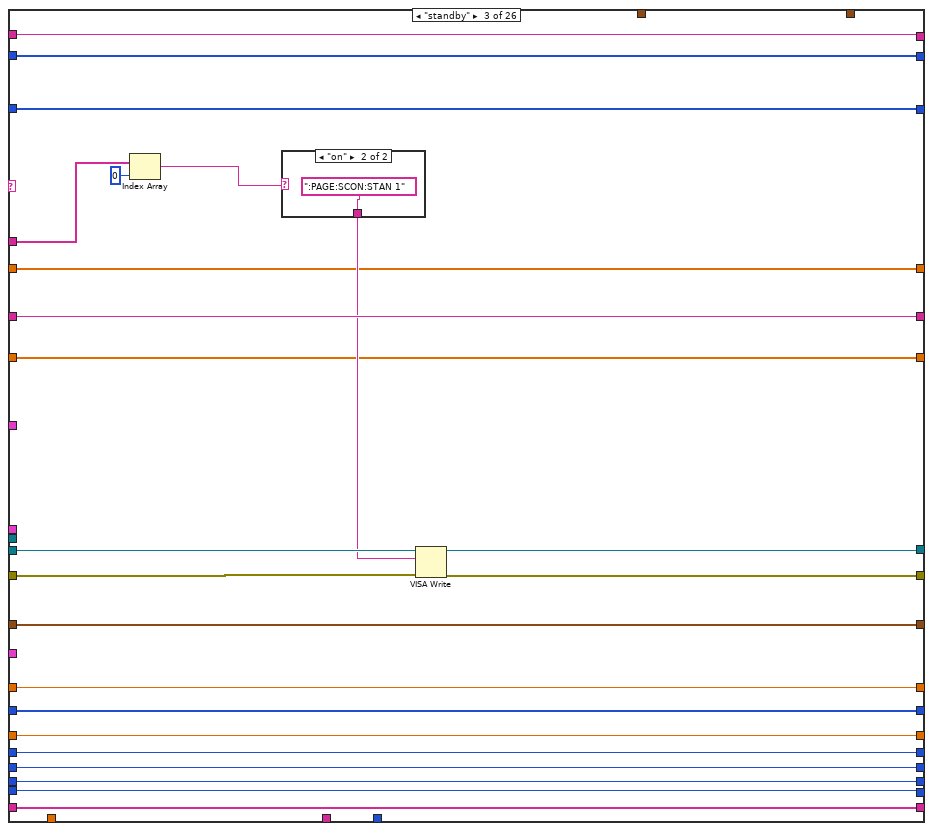
[diagram p6: hidden frame]
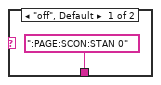
[diagram p7: hidden frame]
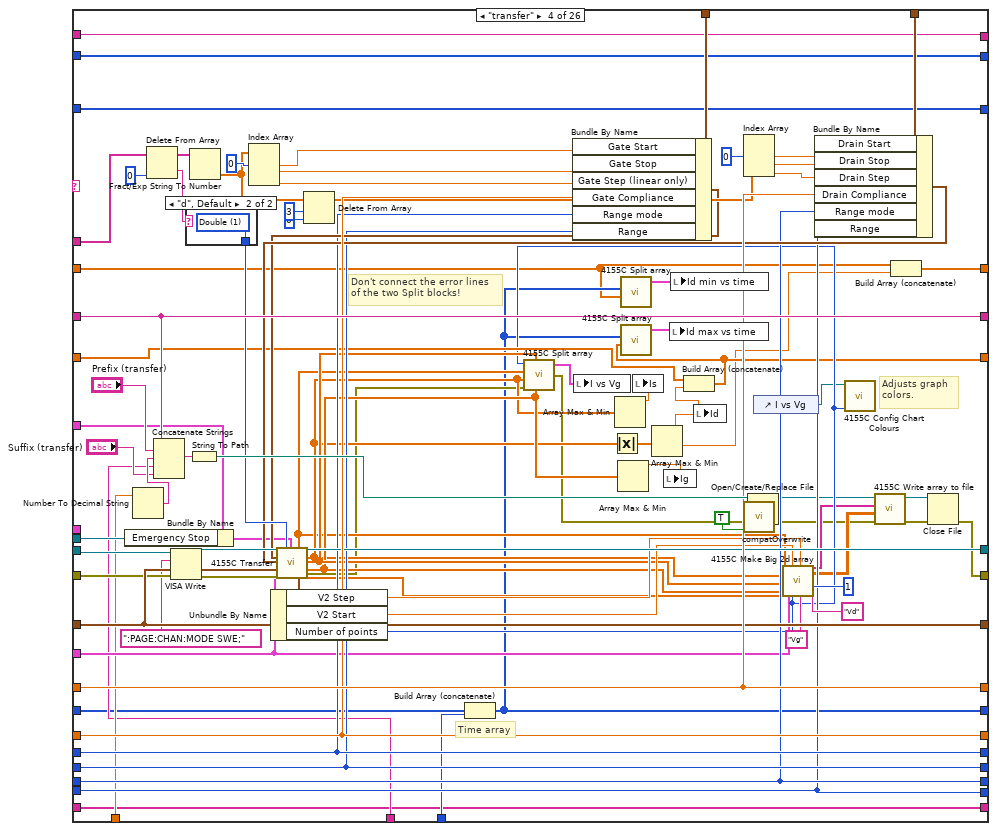
[diagram p8: hidden frame]
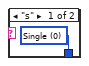
[diagram p9: hidden frame]
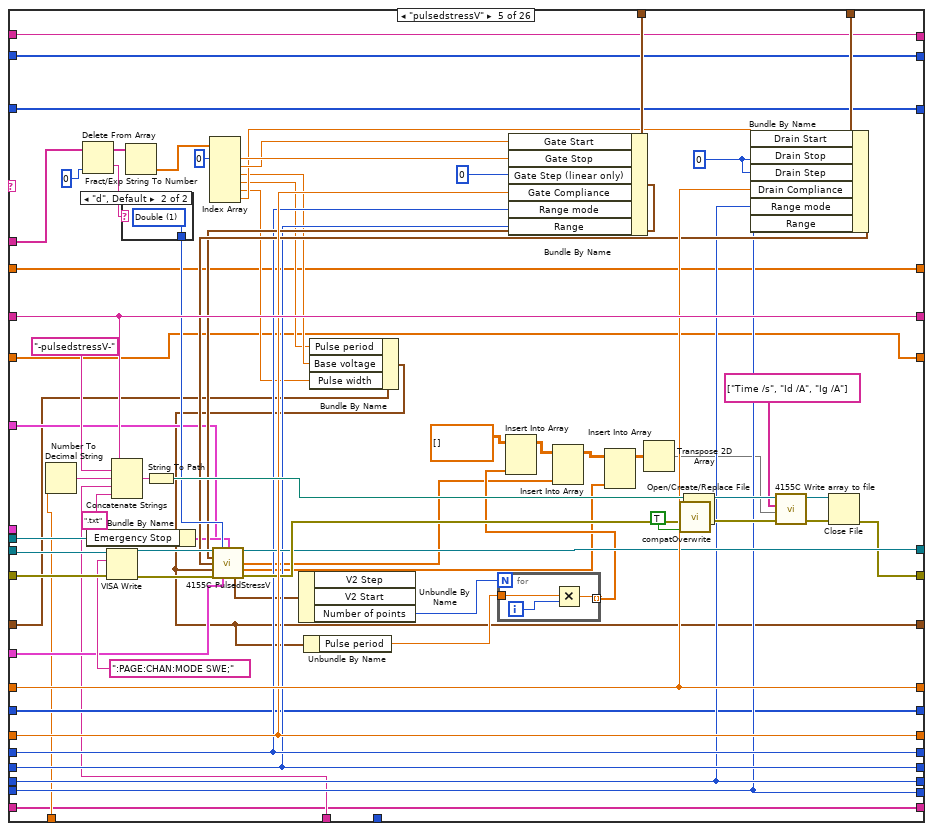
[diagram p10: hidden frame]
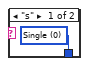
[diagram p11: hidden frame]
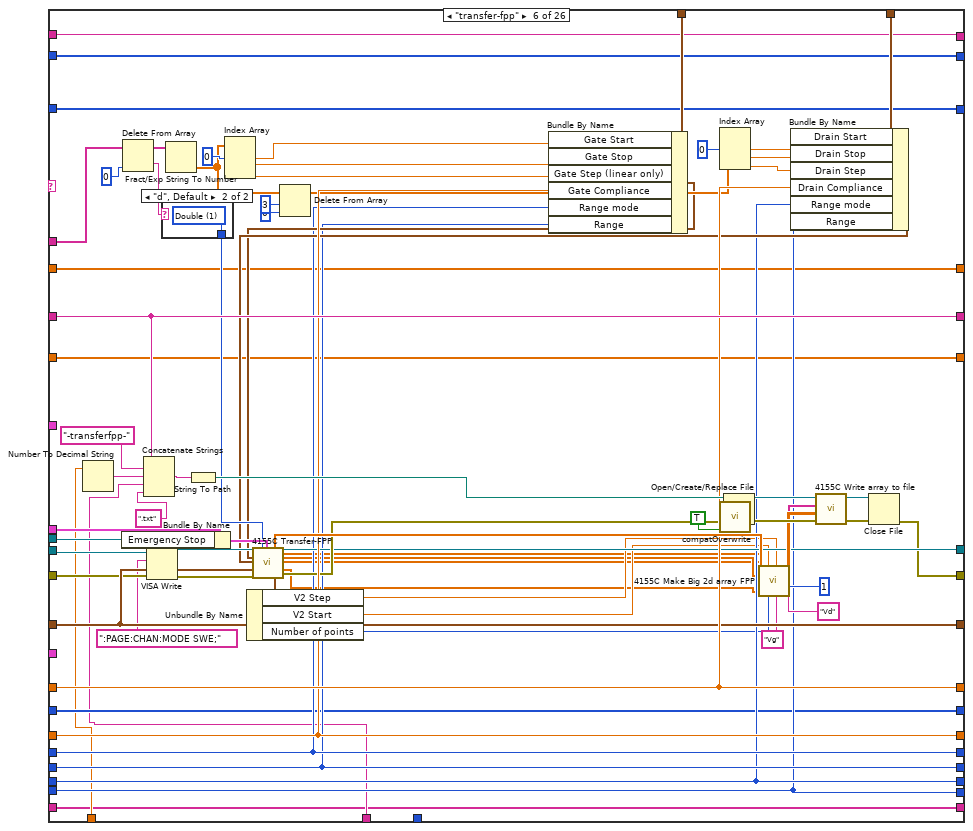
[diagram p12: hidden frame]
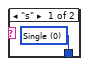
[diagram p13: hidden frame]
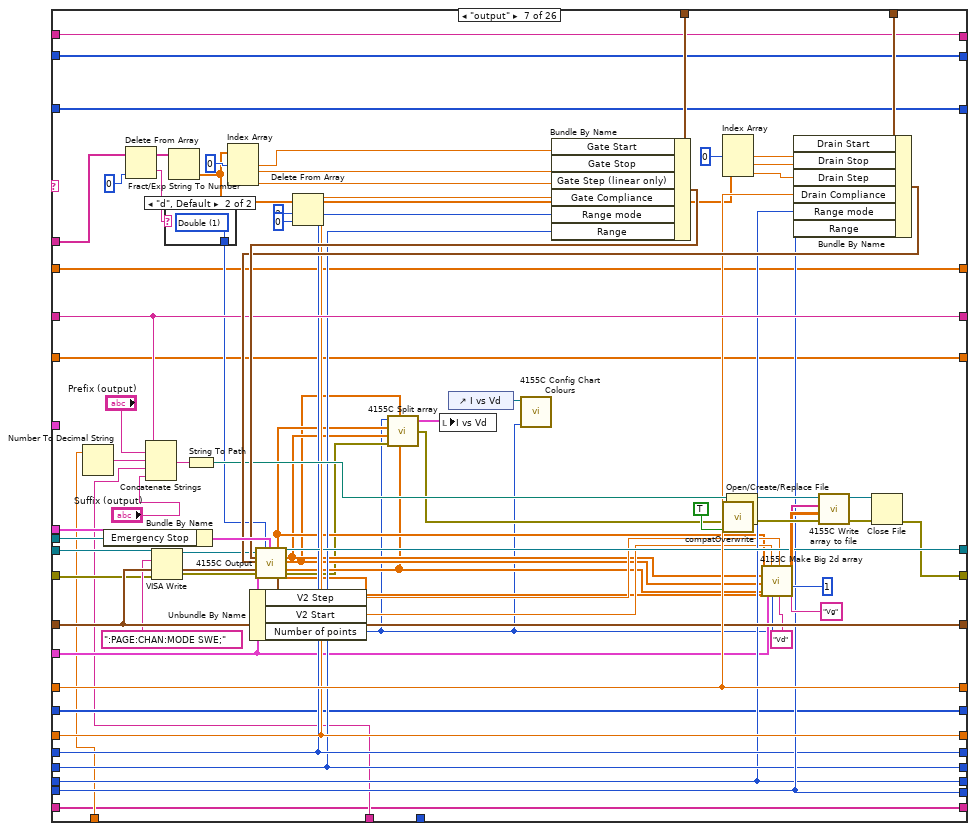
[diagram p14: hidden frame]
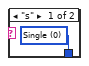
[diagram p15: hidden frame]
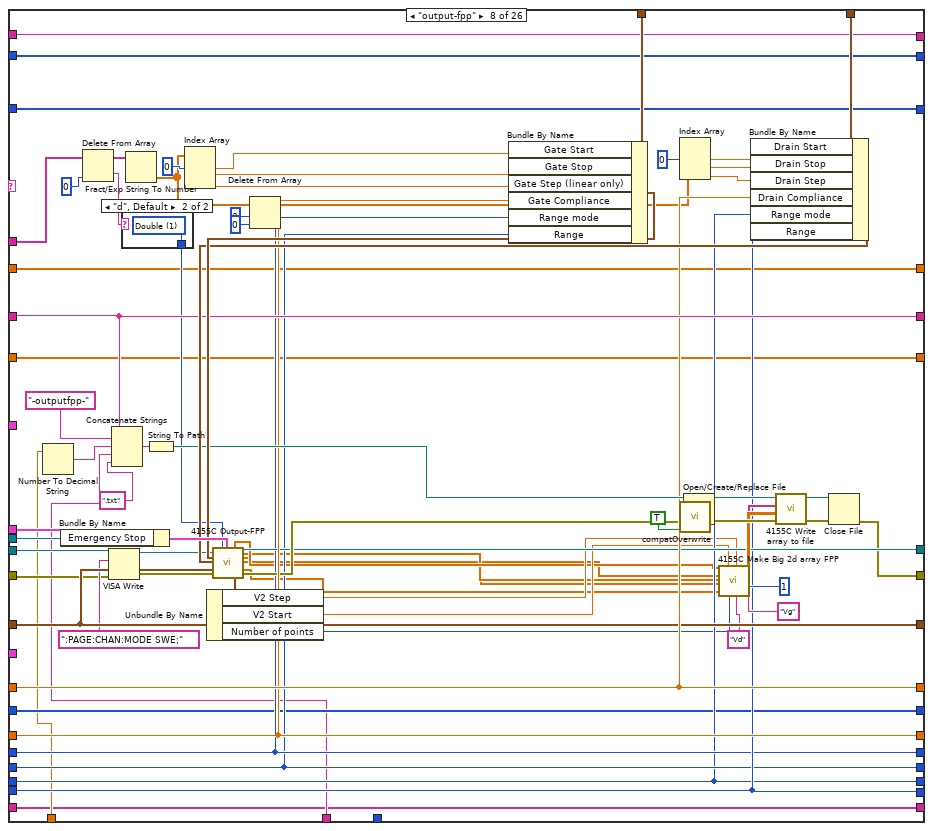
[diagram p16: hidden frame]
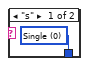
[diagram p17: hidden frame]
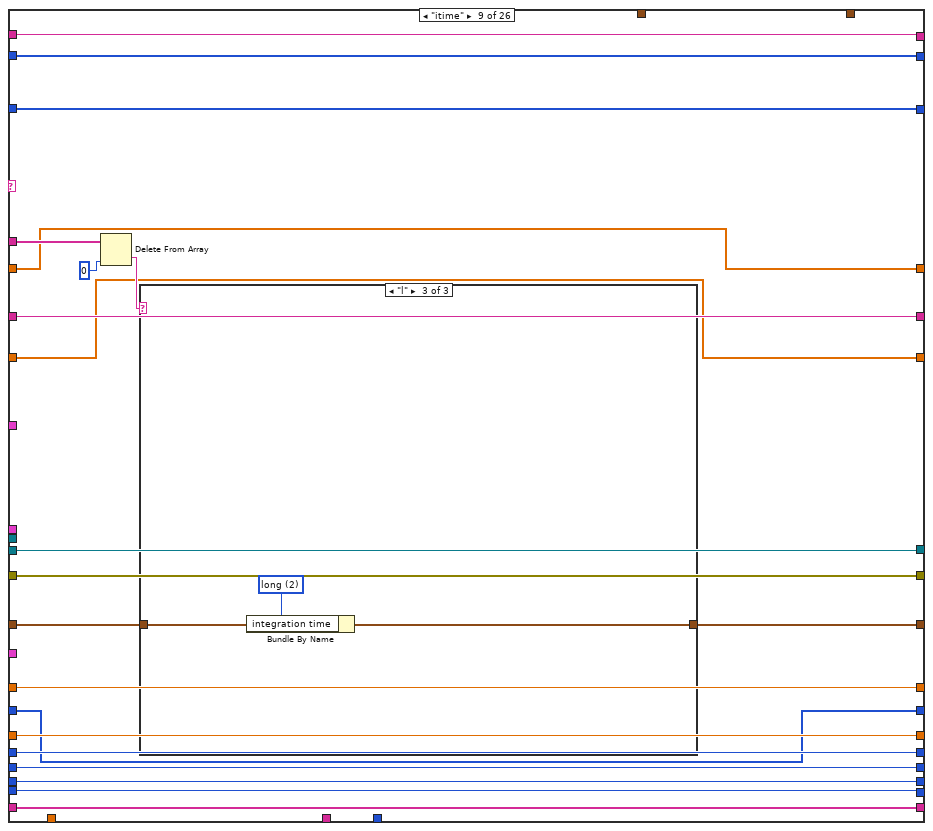
[diagram p18: hidden frame]
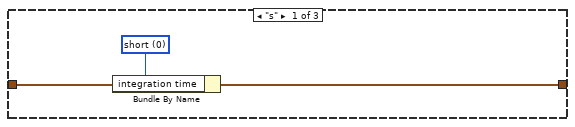
[diagram p19: hidden frame]
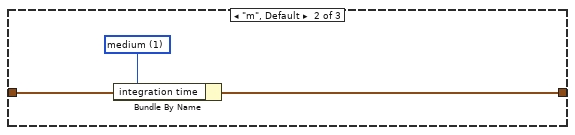
[diagram p20: hidden frame]
diagram:
  w40 = u16 1 items=["Reset All", "Partial reset"] ("Type of reset")
  # "Change from previous version:\n\n- Corrected bug stemming from the fact that the default value of the numeric register is 0. This introduced a 0 in the plunger position and valve position at every SPM command, regardless of what the actual command was."
  # "This is a version specific to the SPM pump."
  # "I add 1 to both the \"total lines\" and the \"line running\" indicators because i and N begin from 0, and the script lines begin from 1."
  # "Bugs:\n\n- Graphs of max and min drain current vs time do not auto-reset between runs. To clear the data you need to restart the vi.\n\n- Do not connect the error message of the Split block if there are unconnected terminals! It will halt the program."
  # "Array size"
  # "%s option converts a spreadsheet string to an array of strings."
  # "0: No of rows of array\n1: No of cols"
  # "Dimitrios Simatos\nv. 4.7"
  # "Changes from original textcontrol.vi:\n\n- Timestamp appears in filename.\n- (Only) transfer and output curves are plotted.\n- Communication with serial port.\n- Can execute any command, as all pattern matching functions were replaced. Previously, commands with special LabVIEW characters could not be executed.\n- Replaced write to file function with write to text file.\n- Replaced while loop with for loop.\n- Replaced 4155C \"Save File\" function and now the vi can save time-dependent variables.\n- Added clock with start time control and various units.\n- Changed filepath in which the program is saved.\n- Added a serial output log that keeps a history.\n- Tab control.\n- Addition of specialized serial read/write file for the SPM OEM pump.\n- Added halt and hard stop."
  # "Search and replace LF with EOL"
  n1 = Equal?(x="integration time", y=u32 0) -> (x = y?=w44:bool)
  n2 = Select(t="Integration time (short)", s=w44, f="Integration time (long)") -> (s? t:f=w48:dbl)
  n3 = call "4155C Get Filename.vi"("error in (no error)"=errorcluster {"status"=FALSE, "code"=0, "source"=""}) -> ("error out"=w35:errorcluster, "path"=w10:path)  [unwired: 2 in, 1 out]
  "Path" <- w10
  n4 = Bundle By Name(cluster="Timings 2", "integration time"="integration time", "Short/Long integration time"=w48, "hold time (sec)"="hold time /s", "delay time (sec)"="delay time /s", "Step Time (0 disables)"="Step delay /s") -> (w33:T6)
  n5 = Path To String(path=w10) -> (string=w11:string)
  n6 = Search and Replace String(replace all?=TRUE ("replace all? (F)"), input string="Program", search string="\n", replace string="\r\n") -> (result string=w23:string)  [unwired: 4 in, 3 out]
  n7 = Match Pattern(string=w11, regular expression=".txt") -> (before substring=w5:string)  [unwired: 1 in, 3 out]
  n8 = Concatenate Strings(w5, "Prefix (script)", ".txt" ("regular expression")) -> (w4:string)
  n9 = call "4155C Initialise.vi"("VISA resource name in"=refnum<visa-resource-name> "GPIB0::14::INSTR", "Reset"="Full Reset", "Type of reset"=w40, "error in (no error)"=w35, "VISA Timeout Value"=u32 10000) -> ("VISA Resource Name out"=w34:refnum<visa-resource-name>, "error out"=w2:errorcluster)
  n10 = Spreadsheet String To Array(delimiter (Tab)="\r\n", format string="%s", spreadsheet string="Program", array type (2D Dbl)="") -> (array=w14:string[][])
  n11 = Array Size(array=w14) -> (size(s)=w18:i32[])
  n12 = String To Path(string=w4) -> (path=w3:path)
  n13 = Write to Text File(file (use dialog)=w3, text=w23, error in=w2) -> (error out=w1:errorcluster)  [unwired: 1 in, 2 out]
  n14 = Index Array(array=w18, index=0) -> (element=w16:i32)
  n15 = for {
    N: w16 -> [w91]
    tunnel: "SMU4" -> [w134]
    shift-left: "Source/Drain Range" -> [w139]
    shift-right: [w135] -> _
    shift-left: "Source/Drain\nRange mode" -> [w140]
    shift-right: [w136] -> _
    shift-left: "Gate Range" -> [w141]
    shift-right: [w137] -> _
    shift-left: "Gate Range\nmode" -> [w142]
    shift-right: [w138] -> _
    shift-left: "Gate: Compliance" -> [w151]
    shift-right: [w147] -> _
    shift-left: "Drain: Compliance" -> [w152]
    shift-right: [w148] -> _
    shift-left: w33 -> [w153]
    shift-right: [w149] -> _
    shift-left: w1 -> [w154]
    shift-right: [w99] -> w9
    shift-left: w34 -> [w155]
    shift-right: [w150] -> _
    shift-left: w5 -> [w156]
    shift-right: [w50] -> _
    tunnel: "Panel Controls 2" -> [w133]
    shift-right: [w103] -> _
    shift-left: _ -> [w132]
    shift-right: [w52] -> _
    shift-left: _ -> [w128]
    tunnel: w14 -> [w126] mode=indexing
    shift-right: [w97] -> _
    shift-left: _ -> [w98]
    shift-right: [w80] -> _
    shift-left: _ -> [w83]
    shift-right: [w53] -> _
    shift-left: _ -> [w73]
    shift-right: [w72] -> _
    shift-left: _ -> [w71]
    shift-right: [w70] -> _
    shift-left: _ -> [w69]
    i -> [w86]
    w54 = "Time /s" ("element")
    # "Valve position"
    # "Valve position"
    # "Pump status"
    # "Absolute plunger position"
    # "Serial port output"
    # "Save serial output log in file."
    # "For loop counter"
    # "<-----Equivalent to the 4155C \"Write\" subvi.----->"
    # "Headers"
    # "Save transfer curves in file."
    # "Filepath and name"
    # "Save time-dependent data."
    # "Use the time offset if your measurements do not start at t=0."
    # "Time"
    # "Rest of elements of command"
    # "Id min"
    # "Id max"
    # "Limit of command arguments (array columns). Raise if needed."
    # "First element of command\n(case select)"
    n16 = Add(x=w91, y=1) -> (x+y=→"Total lines":i32)
    n17 = Add(x=w86, y=1) -> (x+y=→"Line running":i32)
    n18 = Index Array(array=w126, index=0 ("line index")) -> (element=w121:string)
    "Command running:" <- w121
    n19 = Spreadsheet String To Array(delimiter (Tab)=" ", format string="%s", spreadsheet string=w121, array type (2D Dbl)=string[] []) -> (array=w118:string[])
    n20 = control-ref of="Interrupt run"() -> (w146:refnum<vi>)
    n21 = Delete From Array(array=w118, index=0) -> (deleted portion=w119:string, array with subset deleted=w117:string[])  [unwired: 1 in]
    n22 = call "Elapsed Time"("Reset"="Reset", "Auto Reset"="Auto Reset") -> ("Elapsed Time (s)"=w129:dbl)  [unwired: 10 in, 7 out]
    n23 = case shown="0, Default" "Units" {
      tunnel: ["_sec" "_min" "_h"] -> w130
      tunnel: [w157 w161 w164] -> w93
      tunnel: w129 -> [w157 w160 w165]
      frame 0, Default {
      }
      frame 1 {
        n24 = Divide(x=w160, y=60.0) -> (x/y=w161:dbl)
      }
      frame 2 {
        n25 = Divide(x=w165, y=3600.0) -> (x/y=w164:dbl)
      }
    }
    n26 = Add(x=w93, y="Time Offset") -> (x+y=w92:dbl)
    n27 = To Long Integer(number=w92) -> (32bit integer=w127:i32)
    "Elapsed Time" <- w127
    n28 = case shown="\"pump\"" w119 {
      tunnel: w117 -> [w188 w212 w235 w315 w384 w458 w538 w613 w656 w687 w719 w749 w775 w794 _ _ w913 w979 _ w1054 w1103 w1150 w1225 w1292 w1317 w1368]
      tunnel: w156 -> [w183 w208 w233 w322 w391 w466 w545 w621 w645 w676 w711 w742 w769 w787 w811 w858 w891 w961 w997 w1041 w1090 w1138 w1219 w1288 w1319 w1370]
      tunnel: w155 -> [w182 w207 w224 w293 w375 w435 w514 w589 w646 w677 w712 w743 w770 w788 w816 w860 w919 w985 w1001 w1060 w1109 w1156 w1231 w1246 w1323 w1374]
      tunnel: w154 -> [w181 w206 w223 w292 w374 w434 w511 w586 w647 w678 w713 w744 w771 w789 w815 w831 w918 w984 w1000 w1059 w1108 w1155 w1230 w1245 w1322 w1373]
      tunnel: w153 -> [w180 w205 w232 w318 w350 w462 w541 w617 w655 w686 w710 w741 w768 w786 w814 w855 w882 w953 w1006 w1034 w1083 w1131 w1218 w1287 w1324 w1375]
      tunnel: w152 -> [w179 w204 w231 w320 w389 w464 w543 w619 w654 w685 w718 w748 w774 w793 w813 w840 w917 w983 w1009 w1058 w1107 w1154 w1229 w1296 w1325 w1376]
      tunnel: w151 -> [w178 w203 w230 w319 w388 w463 w542 w618 w653 w684 w717 w747 w773 w792 w812 w841 w892 w962 w1008 w1042 w1091 w1139 w1220 w1289 w1327 w1377]
      tunnel: [w182 w207 w222 w317 w386 w460 w540 w615 w646 w677 w712 w743 w770 w788 w816 w860 w883 w935 w999 w1035 w1084 w1132 w1171 w1248 w1323 w1374] -> w150
      tunnel: [w181 w206 w221 w316 w385 w459 w539 w614 w647 w678 w713 w744 w771 w789 w815 w830 w893 w936 w998 w1043 w1092 w1140 w1170 w1247 w1321 w1372] -> w75
      tunnel: [w180 w205 w232 w318 w346 w462 w541 w617 w648 w679 w710 w741 w768 w786 w814 w855 w882 w953 w1006 w1034 w1083 w1131 w1218 w1287 w1324 w1375] -> w149
      tunnel: [w179 w204 w231 w320 w389 w464 w543 w619 w654 w685 w718 w748 w774 w793 w813 w840 w917 w983 w1009 w1058 w1107 w1154 w1229 w1296 w1325 w1376] -> w148
      tunnel: [w178 w203 w230 w319 w388 w463 w542 w618 w653 w684 w717 w747 w773 w792 w812 w841 w892 w962 w1008 w1042 w1091 w1139 w1220 w1289 w1327 w1377] -> w147
      tunnel: [w183 w208 w233 w322 w391 w466 w545 w621 w645 w676 w711 w742 w769 w787 w811 w858 w891 w961 w997 w1041 w1090 w1138 w1219 w1288 w1319 w1370] -> w50
      tunnel: w146 -> [_ _ _ w325 w395 w471 w549 w625 _ _ _ _ _ _ _ _ w888 w958 _ w1040 w1089 w1137 w1191 w1264 _ _]
      tunnel: "Gate" -> [_ _ _ w302 w378 w445 w525 w600 _ _ _ _ _ _ _ _ _ _ _ _ _ _ _ _ _ _]
      tunnel: "Drain 2" -> [_ _ _ w301 w377 w444 w524 w599 _ _ _ _ _ _ _ _ _ _ _ _ _ _ _ _ _ _]
      tunnel: "Panel Controls" -> [_ _ _ _ _ w443 w523 w598 _ _ _ _ _ _ _ _ _ _ _ _ _ _ _ _ _ _]
      tunnel: w142 -> [w177 w202 w229 w286 w368 w428 w509 w584 w652 w683 _ w740 w767 w785 w810 w842 w878 w949 w1002 w1030 w1079 w1127 w1214 w1283 w1328 w1378]
      tunnel: w141 -> [w176 w201 w228 w285 w367 w427 w508 w583 w651 w682 w716 _ w758 w791 w809 w843 w879 w950 w1003 w1031 w1080 w1128 w1215 w1284 w1329 w1379]
      tunnel: w140 -> [w175 w200 w227 w284 w366 w426 w507 w582 w650 w681 w715 w746 w772 _ w808 w844 w880 w951 w1004 w1032 w1081 w1129 w1216 w1285 w1330 w1380]
      tunnel: w139 -> [w174 w199 w226 w283 w365 w425 w510 w585 w649 w680 w714 w745 _ w790 w807 w845 w881 w952 w1005 w1033 w1082 w1130 w1217 w1286 w1331 w1381]
      tunnel: [w177 w202 w229 w286 w368 w428 w509 w584 w652 w683 w709 w740 w767 w785 w810 w842 w878 w949 w1002 w1030 w1079 w1127 w1214 w1283 w1328 w1378] -> w138
      tunnel: [w176 w201 w228 w285 w367 w427 w508 w583 w651 w682 w716 w732 w758 w791 w809 w843 w879 w950 w1003 w1031 w1080 w1128 w1215 w1284 w1329 w1379] -> w137
      tunnel: [w175 w200 w227 w284 w366 w426 w507 w582 w650 w681 w715 w746 w772 w784 w808 w844 w880 w951 w1004 w1032 w1081 w1129 w1216 w1285 w1330 w1380] -> w136
      tunnel: [w174 w199 w226 w283 w365 w425 w510 w585 w649 w680 w714 w745 w759 w790 w807 w845 w881 w952 w1005 w1033 w1082 w1130 w1217 w1286 w1331 w1381] -> w135
      tunnel: w134 -> [_ _ _ w278 w362 _ w503 _ _ _ _ _ _ _ _ _ _ _ _ _ _ _ _ _ _ _]
      tunnel: w133 -> [_ _ _ w276 w361 _ _ _ _ _ _ _ _ _ _ _ _ _ _ _ _ _ _ _ _ _]
      tunnel: [w173 w195 w219 w253 w338 w415 w500 w571 w644 w674 w708 w731 w757 w783 w806 w826 w870 w933 w996 w1019 w1072 w1121 w1168 w1241 w1320 w1371] -> w103
      tunnel: w132 -> [w173 w195 w219 w267 w338 w415 w500 w571 w644 w674 w708 w731 w757 w783 w806 w826 w870 w933 w996 w1019 w1072 w1121 w1168 w1241 w1320 w1371]
      tunnel: w92 -> [_ _ _ w263 w335 w413 w497 w568 _ _ _ _ _ _ _ w824 w868 w930 _ w1016 w1069 w1118 w1165 w1237 _ _]
      tunnel: w130 -> [_ _ _ w260 w334 w411 w496 w567 _ _ _ _ _ _ _ w822 w866 w929 _ w1015 w1068 w1117 w1164 w1238 _ w1339]
      tunnel: w127 -> [_ _ _ w254 _ _ _ _ _ _ _ _ _ _ _ _ _ _ _ _ _ _ _ _ _ w1342]
      tunnel: [w172 w194 w218 w251 w337 w414 w499 w570 w643 w673 w707 w730 w756 w782 w805 w825 w869 w932 w995 w1018 w1071 w1120 w1167 w1240 w1326 w1351] -> w52
      tunnel: w128 -> [w172 w194 w218 w259 w337 w414 w499 w570 w643 w673 w707 w730 w756 w782 w805 w825 w869 w932 w995 w1018 w1071 w1120 w1167 w1240 w1326 w1351]
      tunnel: [w171 w193 w217 w249 w333 w410 w495 w566 w642 w672 w706 w729 w755 w781 w804 w821 w865 w928 w994 w1014 w1067 w1116 w1163 w1236 w1315 w1367] -> w97
      tunnel: w98 -> [w171 w193 w217 w248 w333 w410 w495 w566 w642 w672 w706 w729 w755 w781 w804 w821 w865 w928 w994 w1014 w1067 w1116 w1163 w1236 w1315 w1367]
      tunnel: [w170 w192 w216 w241 w332 w409 w485 w565 w641 w671 w705 w728 w754 w780 w803 w820 w864 w927 w993 w1013 w1066 w1115 w1162 w1235 w1314 w1366] -> w80
      tunnel: w83 -> [w170 w192 w216 w241 w332 w409 w485 w565 w641 w671 w705 w728 w754 w780 w803 w820 w864 w927 w993 w1013 w1066 w1115 w1162 w1235 w1313 w1340]
      tunnel: [w169 w191 w215 w240 w331 w408 w484 w564 w640 w670 w704 w727 w753 w779 w802 w819 w863 w926 w992 w1012 w1065 w1114 w1161 w1234 w1299 w1353] -> w53
      tunnel: w73 -> [w169 w191 w215 w240 w331 w408 w484 w564 w640 w670 w704 w727 w753 w779 w802 w819 w863 w926 w992 w1012 w1065 w1114 w1161 w1234 w1299 w1352]
      tunnel: [w168 w190 w214 w239 w330 w407 w483 w563 w639 w669 w703 w726 w752 w778 w801 w818 w862 w925 w991 w1011 w1064 w1113 w1160 w1233 w1298 w1335] -> w72
      tunnel: w71 -> [w168 w190 w214 w239 w330 w407 w483 w563 w639 w669 w703 w726 w752 w778 w801 w818 w862 w925 w991 w1011 w1064 w1113 w1160 w1233 w1298 w1333]
      tunnel: [w167 w189 w213 w238 w329 w406 w482 w562 w638 w668 w702 w725 w751 w777 w800 w817 w861 w924 w990 w1010 w1063 w1112 w1159 w1232 w1297 w1332] -> w70
      tunnel: w69 -> [w167 w189 w213 w238 w329 w406 w482 w562 w638 w668 w702 w725 w751 w777 w800 w817 w861 w924 w990 w1010 w1063 w1112 w1159 w1232 w1297 w1343]
      frame "wait" {
        n29 = Index Array(array=w188, index=0 ("Index")) -> (element=w186:string)
        n30 = Decimal String To Number(string=w186, default (0L)=u32 0) -> (number=w185:u32)  [unwired: 1 in, 1 out]
        n31 = Wait (ms)(milliseconds to wait=w185) -> ()  [unwired: 1 out]
      }
      frame "wait-min" {
        n32 = Index Array(array=w212, index=0 ("Index")) -> (element=w210:string)
        n33 = Decimal String To Number(string=w210, default (0L)=u32 0) -> (number=w198:u32)  [unwired: 1 in, 1 out]
        n34 = Multiply(x=w198, y=u32 60000) -> (x*y=w197:u32)
        n35 = Wait (ms)(milliseconds to wait=w197) -> ()  [unwired: 1 out]
      }
      frame "standby" {
        n36 = Index Array(array=w235, index=0 ("Index")) -> (element=w225:string)
        n37 = case shown="\"on\"" w225 {
          tunnel: [":PAGE:SCON:STAN 0" ":PAGE:SCON:STAN 1"] -> w220
          frame "off", Default {
          }
          frame "on" {
          }
        }
        n38 = VISA Write(VISA resource name=w224, write buffer=w220, error in (no error)=w223) -> (VISA resource name out=w222:refnum<visa-resource-name>, error out=w221:errorcluster)  [unwired: 1 out]
      }
      frame "transfer" {
        # "Don't connect the error lines\nof the two Split blocks!"
        # "Adjusts graph colors."
        # "Time array"
        n39 = Bundle By Name(cluster=w276, "Emergency Stop"=w325) -> (w277:T2)
        n40 = Number To Decimal String(number=w263) -> (decimal integer string=w262:string)  [unwired: 1 in]
        n41 = Delete From Array(array=w315, index=0 ("Index")) -> (deleted portion=w313:string, array with subset deleted=w312:string[])  [unwired: 1 in]
        n42 = Concatenate Strings(w322, "Prefix (transfer)", w262, w260, "Suffix (transfer)") -> (w324:string)
        n43 = VISA Write(VISA resource name=w293, write buffer=":PAGE:CHAN:MODE SWE;" ("write buffer (\"\")"), error in (no error)=w292) -> (VISA resource name out=w290:refnum<visa-resource-name>, error out=w291:errorcluster)  [unwired: 1 out]
        n44 = case shown="\"d\", Default" w313 {
          tunnel: [w327 w328] -> w311
          frame "s" {
            w327 = u16 0 items=["Single", "Double"] ("sweep mode")
          }
          frame "d", Default {
            w328 = u16 1 items=["Single", "Double"] ("sweep mode")
          }
        }
        n45 = String To Path(string=w324) -> (path=w321:path)
        n46 = Fract/Exp String To Number(string=w312) -> (number=w297:dbl[])  [unwired: 3 in, 1 out]
        n47 = Index Array(array=w297, index #1=0 ("Index")) -> (element #1=w310:dbl, element #2=w309:dbl, element #3=w308:dbl)  [unwired: 2 in]
        n48 = Delete From Array(array=w297, length=3 ("Length"), index=0 ("Index")) -> (array with subset deleted=w295:dbl[])  [unwired: 1 out]
        n49 = Build Array (concatenate)(w259, w254) -> (w251:i32[])
        n50 = Bundle By Name(cluster=w302, "Gate Start"=w310, "Gate Stop"=w309, "Gate Step (linear only)"=w308, "Gate Compliance"=w319, "Range mode"=w286, "Range"=w285) -> (w287:T4)
        n51 = call "4155C Split array.vi"("X data in"=w251, "Y1 data in"=w248) -> ("Array of clusters"=w252:cluster{"Y data in":dbl[], "X data in":dbl[]}[])  [unwired: 5 in, 1 out]
        n52 = local write "Id min vs time"(w252) -> ()
        n53 = Index Array(array=w295, index #1=0 ("Index")) -> (element #1=w305:dbl, element #2=w304:dbl, element #3=w303:dbl)  [unwired: 2 in]
        n54 = call <vilib>:"compatOverwrite.vi"("overwrite (F)"=TRUE) -> ("overwrite?"=w275:T7)
        n55 = control-ref of="I vs Vg"() -> (w264:refnum<vi>)
        n56 = Bundle By Name(cluster=w301, "Drain Start"=w305, "Drain Stop"=w304, "Drain Step"=w303, "Drain Compliance"=w320, "Range mode"=w284, "Range"=w283) -> (w288:T5)
        n57 = call "4155C Transfer.vi"("VISA resource name in"=w290, "Gate"=w287, "Drain"=w288, "Timings"=w318, "error in (no error)"=w291, "SMU4"=w278, "sweep mode"=w311, "Panel Controls"=w277) -> ("VG"=w268:dbl[], "Outparams"=w282:T8, "VISA Resource Name out"=w317:refnum<visa-resource-name>, "IS"=w269:dbl[], "ID"=w274:dbl[], "IG"=w270:dbl[], "error out"=w255:errorcluster, "SMU4"=w279:dbl[])  [unwired: 12 in]
        n58 = Unbundle By Name(w282) -> ("V2 Step"=w281:dbl, "V2 Start"=w280:dbl, "Number of points"=w265:i32)
        n59 = call "4155C Split array.vi"("Number of VAR2 steps"=w265, "Y2 data in"=w274, "X data in"=w268, "Y1 data in"=w269, "Y3 data in"=w270, "error in (no error)"=w255) -> ("Array of clusters"=w258:cluster{"Y data in":dbl[], "X data in":dbl[]}[], "error out"=w256:errorcluster)  [unwired: 1 in]
        n60 = local write "I vs Vg"(w258) -> ()
        n61 = Absolute Value(x=w269) -> (abs(x)=w273:dbl[])
        n62 = Array Max & Min(array=w269) -> (max value=w271:dbl)  [unwired: 3 out]
        n63 = Array Max & Min(array=w270) -> (max value=w272:dbl)  [unwired: 3 out]
        n64 = local write "Is"(w271) -> ()
        n65 = Array Max & Min(array=w273) -> (max value=w266:dbl, min value=w250:dbl)  [unwired: 2 out]
        n66 = local write "Ig"(w272) -> ()
        n67 = Build Array (concatenate)(w267, w266) -> (w253:dbl[])
        n68 = call "4155C Split array.vi"("X data in"=w251, "Y1 data in"=w253) -> ("Array of clusters"=w257:cluster{"Y data in":dbl[], "X data in":dbl[]}[])  [unwired: 5 in, 1 out]
        n69 = local write "Id max vs time"(w257) -> ()
        n70 = local write "Id"(w266) -> ()
        n71 = Open/Create/Replace File(file path (use dialog)=w321, error in=w256, operation (0:open)=w275) -> (refnum out=w246:refnum<file>, error out=w244:errorcluster)  [unwired: 3 in, 1 out]
        n72 = call "4155C Make Big 2d array.vi"("1D Var1"=w268, "1d IS"=w269, "1d ID"=w274, "1d IG"=w270, "1d SMU4"=w279, "SMU4"=w278, "VAR2 START"=w280, "Number of VAR2 steps"=w265, "VAR2 STEP"=w281, "VAR1 Name"="Vg", "Decimal places in header"=i8 1, "VAR2 Name"="Vd") -> ("Header array"=w247:string[], "Data array"=w245:dbl[][])  [unwired: 14 in]
        n73 = call "4155C Config Chart Colours.vi"("Numeric"=w265, "XY Graph 2"=w264) -> ()  [unwired: 6 in]
        n74 = call "4155C Write array to file.vi"("Byte Stream File Refnum"=w246, "Header"=w247, "Data Array"=w245, "error in (no error)"=w244) -> ("dup refnum"=w243:refnum<file>, "error out"=w242:errorcluster)  [unwired: 1 in]
        n75 = Build Array (concatenate)(w248, w250) -> (w249:dbl[])
        n76 = Close File(refnum=w243, error in=w242) -> (error out=w316:errorcluster)  [unwired: 1 out]
      }
      frame "pulsedstressV" {
        w344 = 0
        n77 = Number To Decimal String(number=w335) -> (decimal integer string=w392:string)  [unwired: 1 in]
        n78 = Delete From Array(array=w384, index=0 ("Index")) -> (deleted portion=w382:string, array with subset deleted=w381:string[])  [unwired: 1 in]
        n79 = Bundle By Name(cluster=w361, "Emergency Stop"=w395) -> (w363:T2)
        n80 = VISA Write(VISA resource name=w375, write buffer=":PAGE:CHAN:MODE SWE;" ("write buffer (\"\")"), error in (no error)=w374) -> (VISA resource name out=w372:refnum<visa-resource-name>, error out=w373:errorcluster)  [unwired: 1 out]
        n81 = Concatenate Strings(w391, "-pulsedstressV-" ("Substring"), w392, w334, ".txt" ("Substring")) -> (w394:string)
        n82 = case shown="\"d\", Default" w382 {
          tunnel: [w404 w405] -> w380
          frame "s" {
            w404 = u16 0 items=["Single", "Double"] ("sweep mode")
          }
          frame "d", Default {
            w405 = u16 1 items=["Single", "Double"] ("sweep mode")
          }
        }
        n83 = Fract/Exp String To Number(string=w381) -> (number=w376:dbl[])  [unwired: 3 in, 1 out]
        n84 = String To Path(string=w394) -> (path=w390:path)
        n85 = Index Array(array=w376, index #1=0 ("Index")) -> (element #1=w353:dbl, element #2=w352:dbl, element #3=w349:dbl, element #4=w348:dbl, element #5=w347:dbl, element #6=w351:dbl)  [unwired: 5 in]
        n86 = Bundle By Name(cluster=w350, "Pulse period"=w348, "Base voltage"=w349, "Pulse width"=w347) -> (w346:T6)
        n87 = Unbundle By Name(w346) -> ("Pulse period"=w354:dbl)
        n88 = Bundle By Name(cluster=w378, "Gate Start"=w352, "Gate Stop"=w353, "Gate Step (linear only)"=0, "Gate Compliance"=w388, "Range mode"=w368, "Range"=w367) -> (w369:T4)
        n89 = call <vilib>:"compatOverwrite.vi"("overwrite (F)"=TRUE) -> ("overwrite?"=w339:T7)
        n90 = Bundle By Name(cluster=w377, "Drain Start"=w351, "Drain Stop"=w344, "Drain Step"=w344, "Drain Compliance"=w389, "Range mode"=w366, "Range"=w365) -> (w370:T5)
        n91 = call "4155C PulsedStressV.vi"("VISA resource name in"=w372, "sweep mode"=w380, "Panel Controls"=w363, "Gate"=w369, "Drain"=w370, "Timings"=w346, "error in (no error)"=w373, "SMU4"=w362) -> ("VISA Resource Name out"=w386:refnum<visa-resource-name>, "ID"=w342:dbl[], "IG"=w340:dbl[], "Outparams"=w364:T8, "error out"=w387:errorcluster)  [unwired: 3 in]
        n92 = Unbundle By Name(w364) -> ("Number of points"=w341:i32)  [unwired: 2 out]
        n93 = for {
          N: w341 -> [_]
          tunnel: [w401] -> w343 mode=indexing
          tunnel: w354 -> [w403]
          i -> [w402]
          n94 = Multiply(x=w403, y=w402) -> (x*y=w401:dbl)
        }
        n95 = Insert Into Array(array=dbl[][] [] ("Input Array"), new element=w343) -> (w355:dbl[][])  [unwired: 2 in]
        n96 = Insert Into Array(array=w355, new element=w342) -> (w360:dbl[][])  [unwired: 2 in]
        n97 = Insert Into Array(array=w360, new element=w340) -> (w359:dbl[][])  [unwired: 2 in]
        n98 = Transpose 2D Array(2D array=w359) -> (transposed array=w358:dbl[][])
        n99 = Open/Create/Replace File(file path (use dialog)=w390, error in=w387, operation (0:open)=w339) -> (refnum out=w398:refnum<file>, error out=w399:errorcluster)  [unwired: 3 in, 1 out]
        n100 = call "4155C Write array to file.vi"("Byte Stream File Refnum"=w398, "Header"=string[] ["Time /s", "Id /A", "Ig /A"], "Data Array"=w358, "error in (no error)"=w399) -> ("dup refnum"=w396:refnum<file>, "error out"=w397:errorcluster)  [unwired: 1 in]
        n101 = Close File(refnum=w396, error in=w397) -> (error out=w385:errorcluster)  [unwired: 1 out]
      }
      frame "transfer-fpp" {
        n102 = Number To Decimal String(number=w413) -> (decimal integer string=w467:string)  [unwired: 1 in]
        n103 = Bundle By Name(cluster=w443, "Emergency Stop"=w471) -> (w479:T1)
        n104 = Delete From Array(array=w458, index=0 ("Index")) -> (deleted portion=w456:string, array with subset deleted=w455:string[])  [unwired: 1 in]
        n105 = Concatenate Strings(w466, "-transferfpp-" ("Substring"), w467, w411, ".txt" ("Substring")) -> (w469:string)
        n106 = VISA Write(VISA resource name=w435, write buffer=":PAGE:CHAN:MODE SWE;" ("write buffer (\"\")"), error in (no error)=w434) -> (VISA resource name out=w432:refnum<visa-resource-name>, error out=w433:errorcluster)  [unwired: 1 out]
        n107 = case shown="\"d\", Default" w456 {
          tunnel: [w480 w481] -> w454
          frame "s" {
            w480 = u16 0 items=["Single", "Double"] ("sweep mode")
          }
          frame "d", Default {
            w481 = u16 1 items=["Single", "Double"] ("sweep mode")
          }
        }
        n108 = Fract/Exp String To Number(string=w455) -> (number=w439:dbl[])  [unwired: 3 in, 1 out]
        n109 = String To Path(string=w469) -> (path=w465:path)
        n110 = Index Array(array=w439, index #1=0 ("Index")) -> (element #1=w453:dbl, element #2=w452:dbl, element #3=w451:dbl)  [unwired: 2 in]
        n111 = Delete From Array(array=w439, length=3 ("Length"), index=0 ("Index")) -> (array with subset deleted=w437:dbl[])  [unwired: 1 out]
        n112 = Bundle By Name(cluster=w445, "Gate Start"=w453, "Gate Stop"=w452, "Gate Step (linear only)"=w451, "Gate Compliance"=w463, "Range mode"=w428, "Range"=w427) -> (w429:T4)
        n113 = Index Array(array=w437, index #1=0 ("Index")) -> (element #1=w448:dbl, element #2=w447:dbl, element #3=w446:dbl)  [unwired: 2 in]
        n114 = call <vilib>:"compatOverwrite.vi"("overwrite (F)"=TRUE) -> ("overwrite?"=w416:T7)
        n115 = Bundle By Name(cluster=w444, "Drain Start"=w448, "Drain Stop"=w447, "Drain Step"=w446, "Drain Compliance"=w464, "Range mode"=w426, "Range"=w425) -> (w430:T5)
        n116 = call "4155C Transfer-FPP.vi"("VISA resource name in"=w432, "Gate"=w429, "Drain"=w430, "Timings"=w462, "error in (no error)"=w433, "sweep mode"=w454, "Panel Controls"=w479) -> ("VG"=w470:dbl[], "Outparams"=w424:T8, "VISA Resource Name out"=w460:refnum<visa-resource-name>, "Vprobe2"=w420:dbl[], "ID"=w419:dbl[], "IG"=w418:dbl[], "Vprobe1"=w417:dbl[], "error out"=w461:errorcluster)  [unwired: 13 in]
        n117 = Unbundle By Name(w424) -> ("V2 Step"=w423:dbl, "V2 Start"=w422:dbl, "Number of points"=w421:i32)
        n118 = Open/Create/Replace File(file path (use dialog)=w465, error in=w461, operation (0:open)=w416) -> (refnum out=w476:refnum<file>, error out=w477:errorcluster)  [unwired: 3 in, 1 out]
        n119 = call "4155C Make Big 2d array FPP.vi"("1D Var1"=w470, "1d ID"=w419, "1d Vp2"=w420, "1d IG"=w418, "1d Vp1"=w417, "VAR2 START"=w422, "Number of VAR2 steps"=w421, "VAR2 STEP"=w423, "VAR1 Name"="Vg", "Decimal places in header"=i8 1, "VAR2 Name"="Vd") -> ("Header array"=w472:string[], "Data array"=w473:dbl[][])  [unwired: 15 in]
        n120 = call "4155C Write array to file.vi"("Byte Stream File Refnum"=w476, "Header"=w472, "Data Array"=w473, "error in (no error)"=w477) -> ("dup refnum"=w474:refnum<file>, "error out"=w475:errorcluster)  [unwired: 1 in]
        n121 = Close File(refnum=w474, error in=w475) -> (error out=w459:errorcluster)  [unwired: 1 out]
      }
      frame "output" {
        n122 = Number To Decimal String(number=w497) -> (decimal integer string=w546:string)  [unwired: 1 in]
        n123 = Bundle By Name(cluster=w523, "Emergency Stop"=w549) -> (w559:T1)
        n124 = Delete From Array(array=w538, index=0 ("Index")) -> (deleted portion=w536:string, array with subset deleted=w535:string[])  [unwired: 1 in]
        n125 = Concatenate Strings(w545, "Prefix (output)", w546, w496, "Suffix (output)") -> (w548:string)
        n126 = VISA Write(VISA resource name=w514, write buffer=":PAGE:CHAN:MODE SWE;" ("write buffer (\"\")"), error in (no error)=w511) -> (VISA resource name out=w513:refnum<visa-resource-name>, error out=w512:errorcluster)  [unwired: 1 out]
        n127 = case shown="\"d\", Default" w536 {
          tunnel: [w560 w561] -> w534
          frame "s" {
            w560 = u16 0 items=["Single", "Double"] ("sweep mode")
          }
          frame "d", Default {
            w561 = u16 1 items=["Single", "Double"] ("sweep mode")
          }
        }
        n128 = Fract/Exp String To Number(string=w535) -> (number=w517:dbl[])  [unwired: 3 in, 1 out]
        n129 = String To Path(string=w548) -> (path=w544:path)
        n130 = Index Array(array=w517, index #1=0 ("Index")) -> (element #1=w533:dbl, element #2=w532:dbl, element #3=w531:dbl)  [unwired: 2 in]
        n131 = Delete From Array(array=w517, length=3 ("Length"), index=0 ("Index")) -> (array with subset deleted=w516:dbl[])  [unwired: 1 out]
        n132 = control-ref of="I vs Vd"() -> (w487:refnum<vi>)
        n133 = Bundle By Name(cluster=w525, "Gate Start"=w533, "Gate Stop"=w532, "Gate Step (linear only)"=w531, "Gate Compliance"=w542, "Range mode"=w509, "Range"=w508) -> (w558:T4)
        n134 = Index Array(array=w516, index #1=0 ("Index")) -> (element #1=w528:dbl, element #2=w527:dbl, element #3=w526:dbl)  [unwired: 2 in]
        n135 = call <vilib>:"compatOverwrite.vi"("overwrite (F)"=TRUE) -> ("overwrite?"=w501:T7)
        n136 = Bundle By Name(cluster=w524, "Drain Start"=w528, "Drain Stop"=w527, "Drain Step"=w526, "Drain Compliance"=w543, "Range mode"=w507, "Range"=w510) -> (w557:T5)
        n137 = call "4155C Output.vi"("VISA resource name in"=w513, "Gate"=w558, "Drain"=w557, "Timings"=w541, "error in (no error)"=w512, "SMU4"=w503, "sweep mode"=w534, "Panel controls"=w559) -> ("VD"=w494:dbl[], "Outparams"=w505:T8, "VISA Resource Name out"=w540:refnum<visa-resource-name>, "IS"=w493:dbl[], "ID"=w492:dbl[], "IG"=w491:dbl[], "error out"=w489:errorcluster, "SMU4"=w502:dbl[])  [unwired: 12 in]
        n138 = Unbundle By Name(w505) -> ("V2 Step"=w506:dbl, "V2 Start"=w504:dbl, "Number of points"=w486:i32)
        n139 = call "4155C Split array.vi"("Number of VAR2 steps"=w486, "Y2 data in"=w492, "X data in"=w494, "Y1 data in"=w493, "Y3 data in"=w491, "error in (no error)"=w489) -> ("Array of clusters"=w490:cluster{"Y data in":dbl[], "X data in":dbl[]}[], "error out"=w488:errorcluster)  [unwired: 1 in]
        n140 = local write "I vs Vd"(w490) -> ()
        n141 = call "4155C Config Chart Colours.vi"("Numeric"=w486, "XY Graph 2"=w487) -> ()  [unwired: 6 in]
        n142 = Open/Create/Replace File(file path (use dialog)=w544, error in=w488, operation (0:open)=w501) -> (refnum out=w554:refnum<file>, error out=w555:errorcluster)  [unwired: 3 in, 1 out]
        n143 = call "4155C Make Big 2d array.vi"("1D Var1"=w494, "1d IS"=w493, "1d ID"=w492, "1d IG"=w491, "1d SMU4"=w502, "SMU4"=w503, "VAR2 START"=w504, "Number of VAR2 steps"=w486, "VAR2 STEP"=w506, "VAR1 Name"="Vd", "Decimal places in header"=i8 1, "VAR2 Name"="Vg") -> ("Header array"=w550:string[], "Data array"=w551:dbl[][])  [unwired: 14 in]
        n144 = call "4155C Write array to file.vi"("Byte Stream File Refnum"=w554, "Header"=w550, "Data Array"=w551, "error in (no error)"=w555) -> ("dup refnum"=w552:refnum<file>, "error out"=w553:errorcluster)  [unwired: 1 in]
        n145 = Close File(refnum=w552, error in=w553) -> (error out=w539:errorcluster)  [unwired: 1 out]
      }
      frame "output-fpp" {
        n146 = Number To Decimal String(number=w568) -> (decimal integer string=w622:string)  [unwired: 1 in]
        n147 = Bundle By Name(cluster=w598, "Emergency Stop"=w625) -> (w635:T1)
        n148 = Delete From Array(array=w613, index=0 ("Index")) -> (deleted portion=w611:string, array with subset deleted=w610:string[])  [unwired: 1 in]
        n149 = VISA Write(VISA resource name=w589, write buffer=":PAGE:CHAN:MODE SWE;" ("write buffer (\"\")"), error in (no error)=w586) -> (VISA resource name out=w588:refnum<visa-resource-name>, error out=w587:errorcluster)  [unwired: 1 out]
        n150 = Concatenate Strings(w621, "-outputfpp-" ("Substring"), w622, w567, ".txt" ("Substring")) -> (w624:string)
        n151 = case shown="\"d\", Default" w611 {
          tunnel: [w636 w637] -> w609
          frame "s" {
            w636 = u16 0 items=["Single", "Double"] ("sweep mode")
          }
          frame "d", Default {
            w637 = u16 1 items=["Single", "Double"] ("sweep mode")
          }
        }
        n152 = Fract/Exp String To Number(string=w610) -> (number=w592:dbl[])  [unwired: 3 in, 1 out]
        n153 = String To Path(string=w624) -> (path=w620:path)
        n154 = Index Array(array=w592, index #1=0 ("Index")) -> (element #1=w608:dbl, element #2=w607:dbl, element #3=w606:dbl)  [unwired: 2 in]
        n155 = Delete From Array(array=w592, length=3 ("Length"), index=0 ("Index")) -> (array with subset deleted=w591:dbl[])  [unwired: 1 out]
        n156 = Bundle By Name(cluster=w600, "Gate Start"=w608, "Gate Stop"=w607, "Gate Step (linear only)"=w606, "Gate Compliance"=w618, "Range mode"=w584, "Range"=w583) -> (w634:T4)
        n157 = Index Array(array=w591, index #1=0 ("Index")) -> (element #1=w603:dbl, element #2=w602:dbl, element #3=w601:dbl)  [unwired: 2 in]
        n158 = call <vilib>:"compatOverwrite.vi"("overwrite (F)"=TRUE) -> ("overwrite?"=w572:T7)
        n159 = Bundle By Name(cluster=w599, "Drain Start"=w603, "Drain Stop"=w602, "Drain Step"=w601, "Drain Compliance"=w619, "Range mode"=w582, "Range"=w585) -> (w633:T5)
        n160 = call "4155C Output-FPP.vi"("VISA resource name in"=w588, "Gate"=w634, "Drain"=w633, "Timings"=w617, "error in (no error)"=w587, "sweep mode"=w609, "Panel controls"=w635) -> ("VD"=w577:dbl[], "Outparams"=w580:T8, "VISA Resource Name out"=w615:refnum<visa-resource-name>, "Vprobe2"=w576:dbl[], "ID"=w575:dbl[], "IG"=w574:dbl[], "Vprobe1"=w573:dbl[], "error out"=w616:errorcluster)  [unwired: 13 in]
        n161 = Unbundle By Name(w580) -> ("V2 Step"=w581:dbl, "V2 Start"=w579:dbl, "Number of points"=w578:i32)
        n162 = Open/Create/Replace File(file path (use dialog)=w620, error in=w616, operation (0:open)=w572) -> (refnum out=w630:refnum<file>, error out=w631:errorcluster)  [unwired: 3 in, 1 out]
        n163 = call "4155C Make Big 2d array FPP.vi"("1D Var1"=w577, "1d ID"=w575, "1d Vp2"=w576, "1d IG"=w574, "1d Vp1"=w573, "VAR2 START"=w579, "Number of VAR2 steps"=w578, "VAR2 STEP"=w581, "VAR1 Name"="Vd", "Decimal places in header"=i8 1, "VAR2 Name"="Vg") -> ("Header array"=w626:string[], "Data array"=w627:dbl[][])  [unwired: 15 in]
        n164 = call "4155C Write array to file.vi"("Byte Stream File Refnum"=w630, "Header"=w626, "Data Array"=w627, "error in (no error)"=w631) -> ("dup refnum"=w628:refnum<file>, "error out"=w629:errorcluster)  [unwired: 1 in]
        n165 = Close File(refnum=w628, error in=w629) -> (error out=w614:errorcluster)  [unwired: 1 out]
      }
      frame "itime" {
        n166 = Delete From Array(array=w656, index=0 ("Index")) -> (deleted portion=w657:string)  [unwired: 1 in, 1 out]
        n167 = case shown="\"l\"" w657 {
          tunnel: w655 -> [w661 w663 w666]
          tunnel: [w660 w662 w665] -> w648
          frame "s" {
            w659 = u32 0 items=["short  ", "medium  ", "long  "] ("integration time 2")
            n168 = Bundle By Name(cluster=w661, "integration time"=w659) -> (w660:T6)
          }
          frame "m", Default {
            w664 = u32 1 items=["short  ", "medium  ", "long  "] ("integration time 2")
            n169 = Bundle By Name(cluster=w663, "integration time"=w664) -> (w662:T6)
          }
          frame "l" {
            w667 = u32 2 items=["short  ", "medium  ", "long  "] ("integration time 2")
            n170 = Bundle By Name(cluster=w666, "integration time"=w667) -> (w665:T6)
          }
        }
      }
      frame "pulsed" {
        n171 = Delete From Array(array=w687, index=0 ("Index")) -> (deleted portion=w688:string, array with subset deleted=w675:string[])  [unwired: 1 in]
        n172 = case shown="\"on\", Default" w688 {
          tunnel: w686 -> [w698 w701]
          tunnel: [w697 w700] -> w679
          tunnel: w675 -> [w695 _]
          frame "on", Default {
            w696 = u16 1 items=["Continuous", "Pulsed"] ("sweep method")
            n173 = Fract/Exp String To Number(string=w695) -> (number=w693:dbl[])  [unwired: 3 in, 1 out]
            n174 = Index Array(array=w693, index #1=0 ("Index")) -> (element #1=w692:dbl, element #2=w691:dbl, element #3=w690:dbl)  [unwired: 2 in]
            n175 = Bundle By Name(cluster=w698, "sweep method"=w696, "Pulse period"=w692, "Base voltage"=w691, "Pulse width"=w690) -> (w697:T6)
          }
          frame "off" {
            w699 = u16 0 items=["Continuous", "Pulsed"] ("sweep method")
            n176 = Bundle By Name(cluster=w701, "sweep method"=w699) -> (w700:T6)
          }
        }
      }
      frame "gaterangemode" {
        n177 = Delete From Array(array=w719, index=0 ("Index")) -> (deleted portion=w720:string)  [unwired: 1 in, 1 out]
        n178 = case shown="\"f\"" w720 {
          tunnel: [w722 w723 w724] -> w709
          frame "a", Default {
            w722 = u16 0 items=["Auto", "Limited", "Fixed"] ("Gate Range\nmode 2")
          }
          frame "f" {
            w723 = u16 2 items=["Auto", "Limited", "Fixed"] ("Gate Range\nmode 2")
          }
          frame "l" {
            w724 = u16 1 items=["Auto", "Limited", "Fixed"] ("Gate Range\nmode 2")
          }
        }
      }
      frame "gaterange" {
        (unwired) u8 11 items=["10fA  ", "100fA  ", "1nA  ", "10nA", "100nA", "1uA", "10uA", "100uA", "1mA", "10mA", "100mA", "1A"] ("Gate Range 2")
        n179 = Delete From Array(array=w749, index=0 ("Index")) -> (deleted portion=w739:string)  [unwired: 1 in, 1 out]
        n180 = Scan Value(string=w739, format string="") -> (value=w737:dbl)  [unwired: 1 in, 1 out]
        n181 = Logarithm Base 10(1:w737) -> (0:w736:dbl)
        n182 = Round To Nearest(number=w736) -> (nearest integer value=w735:dbl)
        n183 = Add(x=w735, y=11.0) -> (x+y=w733:dbl)
        n184 = To Unsigned Byte Integer(number=w733) -> (unsigned 8bit integer=w732:u8)
      }
      frame "drainrange" {
        (unwired) u8 11 items=["10fA  ", "100fA  ", "1nA  ", "10nA", "100nA", "1uA", "10uA", "100uA", "1mA", "10mA", "100mA", "1A"] ("Gate Range 2")
        n185 = Delete From Array(array=w775, index=0 ("Index")) -> (deleted portion=w766:string)  [unwired: 1 in, 1 out]
        n186 = Scan Value(string=w766, format string="") -> (value=w764:dbl)  [unwired: 1 in, 1 out]
        n187 = Logarithm Base 10(1:w764) -> (0:w763:dbl)
        n188 = Round To Nearest(number=w763) -> (nearest integer value=w762:dbl)
        n189 = Add(x=w762, y=11.0) -> (x+y=w760:dbl)
        n190 = To Unsigned Byte Integer(number=w760) -> (unsigned 8bit integer=w759:u8)
      }
      frame "drainrangemode" {
        n191 = Delete From Array(array=w794, index=0 ("Index")) -> (deleted portion=w795:string)  [unwired: 1 in, 1 out]
        n192 = case shown="\"f\"" w795 {
          tunnel: [w797 w798 w799] -> w784
          frame "a", Default {
            w797 = u16 0 items=["Auto", "Limited", "Fixed"] ("Gate Range\nmode 2")
          }
          frame "f" {
            w798 = u16 2 items=["Auto", "Limited", "Fixed"] ("Gate Range\nmode 2")
          }
          frame "l" {
            w799 = u16 1 items=["Auto", "Limited", "Fixed"] ("Gate Range\nmode 2")
          }
        }
      }
      frame "Error", Default {
      }
      frame "logfile" {
        n193 = Number To Decimal String(number=w824) -> (decimal integer string=w859:string)  [unwired: 1 in]
        n194 = Concatenate Strings(w858, "logfile" ("Substring"), w859, w822, ".txt" ("Substring")) -> (w856:string)
        n195 = String To Path(string=w856) -> (path=w829:path)
        n196 = Unbundle(w855) -> ("integration time"=w854:u32, "Short/Long integration time"=w853:dbl, "hold time (sec)"=w852:dbl, "delay time (sec)"=w851:dbl, "Step Time (0 disables)"=w850:dbl, "sweep method"=w849:u16, "Pulse period"=w848:dbl, "Base voltage"=w847:dbl, "Pulse width"=w846:dbl)
        n197 = Build Array(w854, w853, w852, w851, w850, w849, w848, w847, w846, w840, w841, w842, w843, w844, w845) -> (w833:dbl[])
        n198 = Insert Into Array(array=dbl[][] [] ("Input Array"), new element=w833) -> (w832:dbl[][])  [unwired: 2 in]
        n199 = call <vilib>:"compatOverwrite.vi"("overwrite (F)"=TRUE) -> ("overwrite?"=w827:T7)
        n200 = Open/Create/Replace File(file path (use dialog)=w829, error in=w831, operation (0:open)=w827) -> (refnum out=w837:refnum<file>, error out=w836:errorcluster)  [unwired: 3 in, 1 out]
        n201 = call "4155C Write array to file.vi"("Byte Stream File Refnum"=w837, "Header"=string[] ["Int Time", "Short/Long Itime", "Hold time", "Delay time", "Step time", "Sweep method", "Pulse period", "Base Voltage", "Pulse width", "Drain compliance", "Gate compliance", "Gate range mode", "Gate range", "S/D range mode", "S/D range"], "Data Array"=w832, "error in (no error)"=w836) -> ("dup refnum"=w839:refnum<file>, "error out"=w838:errorcluster)  [unwired: 1 in]
        n202 = Close File(refnum=w839, error in=w838) -> (error out=w830:errorcluster)  [unwired: 1 out]
      }
      frame "sample" {
        n203 = Number To Decimal String(number=w868) -> (decimal integer string=w916:string)  [unwired: 1 in]
        n204 = Fract/Exp String To Number(string=w913) -> (number=w874:dbl[])  [unwired: 3 in, 1 out]
        n205 = Concatenate Strings(w891, "-sample-" ("Substring"), w916, w866, ".txt" ("Substring")) -> (w914:string)
        n206 = String To Path(string=w914) -> (path=w895:path)
        n207 = Index Array(array=w874, index=0 ("Index")) -> (element=w911:dbl)
        n208 = Index Array(array=w874, index=2 ("Index")) -> (element=w907:dbl)
        n209 = Index Array(array=w874, index=3 ("Index")) -> (element=w876:dbl)
        n210 = Index Array(array=w874, index=4 ("Index")) -> (element=w873:dbl)
        n211 = call "4155C Config Sampling Measurements.vi"("Sampling interval"=w873, "Sample time"=w876, "Display on/off"=TRUE, "Timings"=w882, "Num Points"=w907, "error in (no error)"=w918, "Drain Compliance"=w917, "Gate Compliance"=w892, "VISA session"=w919) -> ("error out"=w920:errorcluster, "dup VISA resource name"=w921:refnum<visa-resource-name>)  [unwired: 1 in]
        n212 = Index Array(array=w874, index=1 ("Index")) -> (element=w908:dbl)
        n213 = call "4155C Take Sample.vi"("Emergency Stop"=w888, "error in (no error)"=w920, "Vd"=w908, "Vg"=w911, "VISA resource name in"=w921) -> ("error out"=w886:errorcluster, "Id"=w923:dbl[], "Ig"=w897:dbl[], "VISA Resource Name out"=w884:refnum<visa-resource-name>, "Is"=w922:dbl[], "Time"=w901:dbl[])  [unwired: 1 in]
        n214 = Insert Into Array(array=dbl[][] [] ("Input Array"), new element=w901) -> (w900:dbl[][])  [unwired: 2 in]
        n215 = Insert Into Array(array=w900, new element=w897) -> (w899:dbl[][])  [unwired: 2 in]
        n216 = Insert Into Array(array=w899, new element=w923) -> (w898:dbl[][])  [unwired: 2 in]
        n217 = VISA Write(VISA resource name=w884, write buffer=":DISP ON" ("write buffer (\"\")"), error in (no error)=w886) -> (VISA resource name out=w883:refnum<visa-resource-name>, error out=w885:errorcluster)  [unwired: 1 out]
        n218 = Insert Into Array(array=w898, new element=w922) -> (w890:dbl[][])  [unwired: 2 in]
        n219 = Transpose 2D Array(2D array=w890) -> (transposed array=w889:dbl[][])
        n220 = call <vilib>:"compatOverwrite.vi"("overwrite (F)"=TRUE) -> ("overwrite?"=w871:T7)
        n221 = Open/Create/Replace File(file path (use dialog)=w895, error in=w885, operation (0:open)=w871) -> (refnum out=w904:refnum<file>, error out=w903:errorcluster)  [unwired: 3 in, 1 out]
        n222 = call "4155C Write array to file.vi"("Byte Stream File Refnum"=w904, "Header"=string[] ["Time /s", "Ig /A", "Id /A", "Is /A"], "Data Array"=w889, "error in (no error)"=w903) -> ("dup refnum"=w906:refnum<file>, "error out"=w905:errorcluster)  [unwired: 1 in]
        n223 = Close File(refnum=w906, error in=w905) -> (error out=w893:errorcluster)  [unwired: 1 out]
      }
      frame "samplei" {
        n224 = Number To Decimal String(number=w930) -> (decimal integer string=w982:string)  [unwired: 1 in]
        n225 = Fract/Exp String To Number(string=w979) -> (number=w946:dbl[])  [unwired: 3 in, 1 out]
        n226 = Concatenate Strings(w961, "-samplei-" ("Substring"), w982, w929, ".txt" ("Substring")) -> (w980:string)
        n227 = String To Path(string=w980) -> (path=w964:path)
        n228 = Index Array(array=w946, index=4 ("Index")) -> (element=w940:dbl)
        n229 = Index Array(array=w946, index=3 ("Index")) -> (element=w941:dbl)
        n230 = Index Array(array=w946, index=1 ("Index")) -> (element=w943:dbl)
        n231 = Index Array(array=w946, index=0 ("Index")) -> (element=w944:dbl)
        n232 = Index Array(array=w946, index=2 ("Index")) -> (element=w942:dbl)
        n233 = call "4155C Config SamplingI Measurements.vi"("Sample time"=w942, "Display on/off"=TRUE, "Timings"=w953, "Num Points"=w943, "error in (no error)"=w984, "Sampling interval"=w941, "VISA session"=w985) -> ("error out"=w986:errorcluster, "dup VISA resource name"=w987:refnum<visa-resource-name>)  [unwired: 3 in]
        n234 = call "4155C Take SampleI.vi"("Emergency Stop"=w958, "error in (no error)"=w986, "Idg 2"=w944, "Vdg compliance 2"=w940, "VISA resource name in"=w987) -> ("error out"=w956:errorcluster, "Idg"=w989:dbl[], "Vdg"=w966:dbl[], "VISA Resource Name out"=w954:refnum<visa-resource-name>, "Is"=w988:dbl[], "Time"=w970:dbl[])  [unwired: 1 in]
        n235 = Insert Into Array(array=dbl[][] [] ("Input Array"), new element=w970) -> (w969:dbl[][])  [unwired: 2 in]
        n236 = Insert Into Array(array=w969, new element=w966) -> (w968:dbl[][])  [unwired: 2 in]
        n237 = Insert Into Array(array=w968, new element=w989) -> (w967:dbl[][])  [unwired: 2 in]
        n238 = VISA Write(VISA resource name=w954, write buffer=":DISP ON" ("write buffer (\"\")"), error in (no error)=w956) -> (VISA resource name out=w939:refnum<visa-resource-name>, error out=w955:errorcluster)  [unwired: 1 out]
        n239 = Insert Into Array(array=w967, new element=w988) -> (w960:dbl[][])  [unwired: 2 in]
        n240 = Transpose 2D Array(2D array=w960) -> (transposed array=w959:dbl[][])
        n241 = call <vilib>:"compatOverwrite.vi"("overwrite (F)"=TRUE) -> ("overwrite?"=w934:T7)
        n242 = Open/Create/Replace File(file path (use dialog)=w964, error in=w955, operation (0:open)=w934) -> (refnum out=w973:refnum<file>, error out=w972:errorcluster)  [unwired: 3 in, 1 out]
        n243 = call "4155C Write array to file.vi"("Byte Stream File Refnum"=w973, "Header"=string[] ["Time /s", "Vdg /V", "Idg /A", "Is /A"], "Data Array"=w959, "error in (no error)"=w972) -> ("dup refnum"=w975:refnum<file>, "error out"=w974:errorcluster)  [unwired: 1 in]
        n244 = Close File(refnum=w975, error in=w974) -> (error out=w937:errorcluster)  [unwired: 1 out]
        n245 = VISA Write(VISA resource name=w939, write buffer=";:PAGE:SCON:STAN OFF;:PAGE:CHAN:VSU2:DIS;" ("write buffer (\"\")"), error in (no error)=w937) -> (VISA resource name out=w935:refnum<visa-resource-name>, error out=w936:errorcluster)  [unwired: 1 out]
      }
      frame "#" {
        n246 = VISA Write(VISA resource name=w1001, write buffer=":DISP ON" ("write buffer (\"\")"), error in (no error)=w1000) -> (VISA resource name out=w999:refnum<visa-resource-name>, error out=w998:errorcluster)  [unwired: 1 out]
      }
      frame "stressV" {
        n247 = Number To Decimal String(number=w1016) -> (decimal integer string=w1057:string)  [unwired: 1 in]
        n248 = Fract/Exp String To Number(string=w1054) -> (number=w1027:dbl[])  [unwired: 3 in, 1 out]
        n249 = Concatenate Strings(w1041, "-stressV-" ("Substring"), w1057, w1015, ".txt" ("Substring")) -> (w1055:string)
        n250 = String To Path(string=w1055) -> (path=w1045:path)
        n251 = Index Array(array=w1027, index=3 ("Index")) -> (element=w1024:dbl)
        n252 = Index Array(array=w1027, index=1 ("Index")) -> (element=w1022:dbl)
        n253 = Index Array(array=w1027, index=0 ("Index")) -> (element=w1021:dbl)
        n254 = Index Array(array=w1027, index=4 ("Index")) -> (element=w1026:dbl)
        n255 = Index Array(array=w1027, index=2 ("Index")) -> (element=w1023:dbl)
        n256 = call "4155C Config V Stress.vi"("VISA session"=w1060, "ID compliance"=w1024, "VD"=w1022, "VG"=w1021, "IG compliance"=w1023, "error in (no error)"=w1059, "Display on/off"=TRUE) -> ("dup VISA resource name"=w1062:refnum<visa-resource-name>, "error out"=w1061:errorcluster)
        n257 = call "4155C Apply Stress.vi"("error in (no error)"=w1061, "Duration"=w1026, "Emergency Stop"=w1040, "VISA resource name in"=w1062) -> ("error out"=w1038:errorcluster, "VISA Resource Name out"=w1036:refnum<visa-resource-name>)
        n258 = VISA Write(VISA resource name=w1036, write buffer=":DISP ON" ("write buffer (\"\")"), error in (no error)=w1038) -> (VISA resource name out=w1035:refnum<visa-resource-name>, error out=w1037:errorcluster)  [unwired: 1 out]
        n259 = call <vilib>:"compatOverwrite.vi"("overwrite (F)"=TRUE) -> ("overwrite?"=w1020:T7)
        n260 = Open/Create/Replace File(file path (use dialog)=w1045, error in=w1037, operation (0:open)=w1020) -> (refnum out=w1048:refnum<file>, error out=w1047:errorcluster)  [unwired: 3 in, 1 out]
        n261 = call "4155C Write array to file.vi"("Byte Stream File Refnum"=w1048, "Header"=string[] ["V stress completed successfully", ""], "error in (no error)"=w1047) -> ("dup refnum"=w1050:refnum<file>, "error out"=w1049:errorcluster)  [unwired: 2 in]
        n262 = Close File(refnum=w1050, error in=w1049) -> (error out=w1043:errorcluster)  [unwired: 1 out]
      }
      frame "stressI" {
        n263 = Number To Decimal String(number=w1069) -> (decimal integer string=w1106:string)  [unwired: 1 in]
        n264 = Fract/Exp String To Number(string=w1103) -> (number=w1078:dbl[])  [unwired: 3 in, 1 out]
        n265 = Concatenate Strings(w1090, "-stressI-" ("Substring"), w1106, w1068, ".txt" ("Substring")) -> (w1104:string)
        n266 = String To Path(string=w1104) -> (path=w1094:path)
        n267 = Index Array(array=w1078, index=1 ("Index")) -> (element=w1074:dbl)
        n268 = Index Array(array=w1078, index=0 ("Index")) -> (element=w1075:dbl)
        n269 = call "4155C Config I Stress.vi"("VISA session"=w1109, "IDG"=w1075, "VDG compliance"=w1074, "error in (no error)"=w1108, "Display on/off"=TRUE) -> ("dup VISA resource name"=w1111:refnum<visa-resource-name>, "error out"=w1110:errorcluster)
        n270 = Index Array(array=w1078, index=2 ("Index")) -> (element=w1076:dbl)
        n271 = call "4155C Apply Stress.vi"("error in (no error)"=w1110, "Duration"=w1076, "Emergency Stop"=w1089, "VISA resource name in"=w1111) -> ("error out"=w1087:errorcluster, "VISA Resource Name out"=w1085:refnum<visa-resource-name>)
        n272 = VISA Write(VISA resource name=w1085, write buffer=":DISP ON" ("write buffer (\"\")"), error in (no error)=w1087) -> (VISA resource name out=w1084:refnum<visa-resource-name>, error out=w1086:errorcluster)  [unwired: 1 out]
        n273 = call <vilib>:"compatOverwrite.vi"("overwrite (F)"=TRUE) -> ("overwrite?"=w1073:T7)
        n274 = Open/Create/Replace File(file path (use dialog)=w1094, error in=w1086, operation (0:open)=w1073) -> (refnum out=w1097:refnum<file>, error out=w1096:errorcluster)  [unwired: 3 in, 1 out]
        n275 = call "4155C Write array to file.vi"("Byte Stream File Refnum"=w1097, "Header"=string[] ["I stress completed successfully", ""], "error in (no error)"=w1096) -> ("dup refnum"=w1099:refnum<file>, "error out"=w1098:errorcluster)  [unwired: 2 in]
        n276 = Close File(refnum=w1099, error in=w1098) -> (error out=w1092:errorcluster)  [unwired: 1 out]
      }
      frame "vsu2pulse" {
        n277 = Number To Decimal String(number=w1118) -> (decimal integer string=w1153:string)  [unwired: 1 in]
        n278 = Fract/Exp String To Number(string=w1150) -> (number=w1126:dbl[])  [unwired: 3 in, 1 out]
        n279 = Concatenate Strings(w1138, "-vsu2-" ("Substring"), w1153, w1117, ".txt" ("Substring")) -> (w1151:string)
        n280 = String To Path(string=w1151) -> (path=w1142:path)
        n281 = Index Array(array=w1126, index=1 ("Index")) -> (element=w1125:dbl)
        n282 = Index Array(array=w1126, index=0 ("Index")) -> (element=w1123:dbl)
        n283 = call "4155C Config VSU2 Stress.vi"("error in (no error)"=w1155, "VSU2"=w1123, "Display on/off"=TRUE, "VISA session"=w1156) -> ("error out"=w1157:errorcluster, "dup VISA resource name"=w1158:refnum<visa-resource-name>)
        n284 = call "4155C Apply Stress.vi"("error in (no error)"=w1157, "Duration"=w1125, "Emergency Stop"=w1137, "VISA resource name in"=w1158) -> ("error out"=w1135:errorcluster, "VISA Resource Name out"=w1133:refnum<visa-resource-name>)
        n285 = VISA Write(VISA resource name=w1133, write buffer=":DISP ON" ("write buffer (\"\")"), error in (no error)=w1135) -> (VISA resource name out=w1132:refnum<visa-resource-name>, error out=w1134:errorcluster)  [unwired: 1 out]
        n286 = call <vilib>:"compatOverwrite.vi"("overwrite (F)"=TRUE) -> ("overwrite?"=w1122:T7)
        n287 = Open/Create/Replace File(file path (use dialog)=w1142, error in=w1134, operation (0:open)=w1122) -> (refnum out=w1145:refnum<file>, error out=w1144:errorcluster)  [unwired: 3 in, 1 out]
        n288 = call "4155C Write array to file.vi"("Byte Stream File Refnum"=w1145, "Header"=string[] ["VSU2 pulse completed successfully", ""], "error in (no error)"=w1144) -> ("dup refnum"=w1147:refnum<file>, "error out"=w1146:errorcluster)  [unwired: 2 in]
        n289 = Close File(refnum=w1147, error in=w1146) -> (error out=w1140:errorcluster)  [unwired: 1 out]
      }
      frame "sample-fpp" {
        w1176 = string[] ["Time /s", "Id VgVd /A", "Ig VgVd /A", "Vp1 VgVd /V", "Vp2 VgVd /V"] ("Header")
        w1180 = "%d" ("format string")
        n290 = Number To Decimal String(number=w1165) -> (decimal integer string=w1228:string)  [unwired: 1 in]
        n291 = Fract/Exp String To Number(string=w1225) -> (number=w1213:dbl[])  [unwired: 3 in, 1 out]
        n292 = Concatenate Strings(w1219, "-samplefpp-" ("Substring"), w1228, w1164, ".txt" ("Substring")) -> (w1226:string)
        n293 = String To Path(string=w1226) -> (path=w1188:path)
        n294 = Index Array(array=w1213, index=0 ("Index")) -> (element=w1174:dbl)
        n295 = Index Array(array=w1213, index=1 ("Index")) -> (element=w1173:dbl)
        n296 = Index Array(array=w1213, index=2 ("Index")) -> (element=w1221:dbl)
        n297 = Index Array(array=w1213, index=3 ("Index")) -> (element=w1211:dbl)
        n298 = call "4155C Config Sampling Measurements FPP.vi"("VISA session"=w1231, "Num Points"=w1221, "Vg"=w1174, "Display on/off"=TRUE, "Gate Compliance"=w1220, "Drain Compliance"=w1229, "Standby"="Standby", "error in (no error)"=w1230, "Timings"=w1218, "Vd"=w1173, "Sample time"=w1211) -> ("dup VISA resource name"=w1190:refnum<visa-resource-name>, "error out"=w1189:errorcluster)  [unwired: 3 in]
        n299 = Number To Decimal String(number=w1174) -> (decimal integer string=w1200:string)  [unwired: 1 in]
        n300 = call "4155C Take Sample FPP.vi"("VISA resource name in"=w1190, "error in (no error)"=w1189, "Emergency Stop"=w1191) -> ("Time"=w1195:dbl[], "Vp1"=w1205:dbl[], "VISA Resource Name out"=w1171:refnum<visa-resource-name>, "Ig"=w1193:dbl[], "Id"=w1194:dbl[], "Vp2"=w1203:dbl[], "error out"=w1192:errorcluster)  [unwired: 10 in]
        n301 = Insert Into Array(array=dbl[][] [] ("Input Array"), new element=w1195) -> (w1209:dbl[][])  [unwired: 2 in]
        n302 = Number To Decimal String(number=w1173) -> (decimal integer string=w1198:string)  [unwired: 1 in]
        n303 = Insert Into Array(array=w1209, new element=w1194) -> (w1208:dbl[][])  [unwired: 2 in]
        n304 = Concatenate Strings("(Vg = " ("Substring"), w1200, "V, Vd = " ("Substring"), w1198, "V)" ("Substring")) -> (w1196:string)
        n305 = Insert Into Array(array=w1208, new element=w1193) -> (w1207:dbl[][])  [unwired: 2 in]
        n306 = Insert Into Array(array=w1207, new element=w1205) -> (w1204:dbl[][])  [unwired: 2 in]
        n307 = Insert Into Array(array=w1204, new element=w1203) -> (w1172:dbl[][])  [unwired: 2 in]
        n308 = call <vilib>:"compatOverwrite.vi"("overwrite (F)"=TRUE) -> ("overwrite?"=w1169:T7)
        n309 = Open/Create/Replace File(file path (use dialog)=w1188, error in=w1192, operation (0:open)=w1169) -> (refnum out=w1185:refnum<file>, error out=w1186:errorcluster)  [unwired: 3 in, 1 out]
        n310 = Array To Spreadsheet String(array=w1176, 3:w1180) -> (spreadsheet string=w1182:string)  [unwired: 1 in]
        n311 = Transpose 2D Array(2D array=w1172) -> (transposed array=w1202:dbl[][])
        n312 = Search and Replace String(replace all?=TRUE ("replace all? (F)"), input string=w1182, search string="VgVd", replace string=w1196) -> (result string=w1178:string)  [unwired: 4 in, 3 out]
        n313 = Spreadsheet String To Array(format string=w1180, spreadsheet string=w1178, array type (2D Dbl)=w1176) -> (array=w1177:string[])  [unwired: 1 in]
        n314 = call "4155C Write array to file.vi"("Byte Stream File Refnum"=w1185, "Header"=w1177, "Data Array"=w1202, "error in (no error)"=w1186) -> ("dup refnum"=w1183:refnum<file>, "error out"=w1184:errorcluster)  [unwired: 1 in]
        n315 = Close File(refnum=w1183, error in=w1184) -> (error out=w1170:errorcluster)  [unwired: 1 out]
      }
      frame "resample-fpp" {
        w1251 = string[] ["Time /s", "Id VgVd /A", "Ig VgVd /A", "Vp1 VgVd /V", "Vp2 VgVd /V"] ("Header")
        w1255 = "%d" ("format string")
        n316 = Number To Decimal String(number=w1237) -> (decimal integer string=w1295:string)  [unwired: 1 in]
        n317 = Fract/Exp String To Number(string=w1292) -> (number=w1244:dbl[])  [unwired: 3 in, 1 out]
        n318 = Concatenate Strings(w1288, "-resamplefpp-" ("Substring"), w1295, w1238, ".txt" ("Substring")) -> (w1293:string)
        n319 = String To Path(string=w1293) -> (path=w1263:path)
        n320 = Index Array(array=w1244, index=0 ("Index")) -> (element=w1250:dbl)
        n321 = Index Array(array=w1244, index=1 ("Index")) -> (element=w1249:dbl)
        n322 = Number To Decimal String(number=w1250) -> (decimal integer string=w1273:string)  [unwired: 1 in]
        n323 = call "4155C Take Sample FPP.vi"("VISA resource name in"=w1246, "error in (no error)"=w1245, "Emergency Stop"=w1264) -> ("Time"=w1268:dbl[], "Vp1"=w1278:dbl[], "VISA Resource Name out"=w1248:refnum<visa-resource-name>, "Ig"=w1266:dbl[], "Id"=w1267:dbl[], "Vp2"=w1276:dbl[], "error out"=w1265:errorcluster)  [unwired: 10 in]
        n324 = Insert Into Array(array=dbl[][] [] ("Input Array"), new element=w1268) -> (w1282:dbl[][])  [unwired: 2 in]
        n325 = Number To Decimal String(number=w1249) -> (decimal integer string=w1271:string)  [unwired: 1 in]
        n326 = Insert Into Array(array=w1282, new element=w1267) -> (w1281:dbl[][])  [unwired: 2 in]
        n327 = Concatenate Strings("(Vg = " ("Substring"), w1273, "V, Vd = " ("Substring"), w1271, "V)" ("Substring")) -> (w1269:string)
        n328 = Insert Into Array(array=w1281, new element=w1266) -> (w1280:dbl[][])  [unwired: 2 in]
        n329 = Insert Into Array(array=w1280, new element=w1278) -> (w1277:dbl[][])  [unwired: 2 in]
        n330 = Insert Into Array(array=w1277, new element=w1276) -> (w1243:dbl[][])  [unwired: 2 in]
        n331 = call <vilib>:"compatOverwrite.vi"("overwrite (F)"=TRUE) -> ("overwrite?"=w1242:T7)
        n332 = Open/Create/Replace File(file path (use dialog)=w1263, error in=w1265, operation (0:open)=w1242) -> (refnum out=w1260:refnum<file>, error out=w1261:errorcluster)  [unwired: 3 in, 1 out]
        n333 = Array To Spreadsheet String(array=w1251, 3:w1255) -> (spreadsheet string=w1257:string)  [unwired: 1 in]
        n334 = Transpose 2D Array(2D array=w1243) -> (transposed array=w1275:dbl[][])
        n335 = Search and Replace String(replace all?=TRUE ("replace all? (F)"), input string=w1257, search string="VgVd", replace string=w1269) -> (result string=w1253:string)  [unwired: 4 in, 3 out]
        n336 = Spreadsheet String To Array(format string=w1255, spreadsheet string=w1253, array type (2D Dbl)=w1251) -> (array=w1252:string[])  [unwired: 1 in]
        n337 = call "4155C Write array to file.vi"("Byte Stream File Refnum"=w1260, "Header"=w1252, "Data Array"=w1275, "error in (no error)"=w1261) -> ("dup refnum"=w1258:refnum<file>, "error out"=w1259:errorcluster)  [unwired: 1 in]
        n338 = Close File(refnum=w1258, error in=w1259) -> (error out=w1247:errorcluster)  [unwired: 1 out]
      }
      frame "serial" {
        n339 = local read "Enable Termination\nChar (T)"() -> (w1310:bool)
        n340 = local read "Termination char\n(0xA = '\\n' = LF)\n(0xD = '\\r' = CR)"() -> (w1309:u8)
        n341 = Index Array(array=w1317, index=0 ("Index")) -> (element=w1316:string)
        n342 = local read "parity"() -> (w1300:u16)
        n343 = local read "Delay before read (ms)"() -> (w1311:u32)
        n344 = local read "byte count"() -> (w1308:u32)
        n345 = local read "Timeout (ms)"() -> (w1307:u32)
        n346 = local read "VISA resource name"() -> (w1304:refnum<visa-resource-name>)
        n347 = local read "baud rate"() -> (w1303:u32)
        n348 = local read "Serial End Mode for Reads"() -> (w1302:u16)
        n349 = local read "data bits"() -> (w1301:u16)
        n350 = local read "stop bits"() -> (w1306:u16)
        n351 = local read "flow control"() -> (w1305:u16)
        n352 = call "Serial write and read v0.5.vi"("Delay before read (ms)"=w1311, "Termination char\n(0xA = '\\n' = LF)\n(0xD = '\\r' = CR)"=w1309, "Enable Termination\nChar (T)"=w1310, "parity"=w1300, "stop bits"=w1306, "string to write"=w1316, "flow control"=w1305, "byte count"=w1308, "Serial Settings:Serial End Mode for Reads"=w1302, "Timeout (ms)"=w1307, "error in (no error)"=w1322, "VISA resource name"=w1304, "baud rate"=w1303, "data bits"=w1301) -> ("Serial port output"=w1312:string, "error out"=w1321:errorcluster)
        n353 = Build Array (concatenate)(w1312, w1313) -> (w1314:string[])
      }
      frame "pump" {
        # "Absolute plunger position"
        # "Remove \"_\""
        # "Check if hard stop is pressed."
        # "Check if halt is pressed."
        # "Check if pump is idle. Else halt."
        n354 = local read "Hard stop pump"() -> (w1347:bool)
        n355 = local read "Halt pump"() -> (w1350:bool)
        n356 = local read "Enable Termination\nChar (T)"() -> (w1364:bool)
        n357 = local read "Termination char\n(0xA = '\\n' = LF)\n(0xD = '\\r' = CR)"() -> (w1363:u8)
        n358 = Index Array(array=w1368, index=0 ("Index")) -> (element=w1345:string)
        n359 = case shown="\"Initialization\"" w1343 {
          tunnel: w1345 -> [w1395 _ w1397 w1398 w1399 w1400 _ _ w1403 w1404 _]
          tunnel: [w1395 "/1H" w1397 w1398 w1399 w1400 "/1H" "/1H" w1403 w1404 "/1H"] -> w1344
          frame "No error", Default {
          }
          frame "Initialization" {
          }
          frame "Invalid command" {
          }
          frame "Invalid operand" {
          }
          frame "Device not initialized" {
          }
          frame "Internal failure" {
          }
          frame "Plunger overload" {
          }
          frame "Valve overload" {
          }
          frame "Plunger move not allowed" {
          }
          frame "A/D converter failure" {
          }
          frame "Command overflow" {
          }
        }
        n360 = case shown="True" w1350 {
          tunnel: [w1409 "/1H"] -> w1349
          tunnel: w1344 -> [w1409 _]
          frame False {
          }
          frame True {
            n361 = local write "Halt pump"(FALSE) -> ()
          }
        }
        n362 = case shown="True" w1347 {
          tunnel: [w1406 "/1T"] -> w1348
          tunnel: w1349 -> [w1406 _]
          frame False {
          }
          frame True {
            n363 = local write "Hard stop pump"(FALSE) -> ()
          }
        }
        n364 = local read "Serial End Mode for Reads"() -> (w1356:u16)
        n365 = local read "flow control"() -> (w1359:u16)
        n366 = local read "stop bits"() -> (w1360:u16)
        n367 = local read "parity"() -> (w1354:u16)
        n368 = local read "Delay before read (ms)"() -> (w1365:u32)
        n369 = local read "byte count"() -> (w1362:u32)
        n370 = local read "Timeout (ms)"() -> (w1361:u32)
        n371 = local read "VISA resource name"() -> (w1358:refnum<visa-resource-name>)
        n372 = local read "baud rate"() -> (w1357:u32)
        n373 = local read "data bits"() -> (w1355:u16)
        n374 = String Subset(string=w1339, offset (0)=1) -> (substring=w1337:string)  [unwired: 1 in]
        n375 = call "SPM Pump v0.5.vi"("Termination char\n(0xA = '\\n' = LF)\n(0xD = '\\r' = CR)"=w1363, "Enable Termination\nChar (T)"=w1364, "Timeout (ms)"=w1361, "Serial Settings:Serial End Mode for Reads"=w1356, "byte count"=w1362, "Delay before read (ms)"=w1365, "Time <input>"=w1342, "error in (no error)"=w1373, "Serial port input"=w1348, "VISA resource name"=w1358, "parity"=w1354, "baud rate"=w1357, "stop bits"=w1360, "data bits"=w1355, "flow control"=w1359, "Time units <input>"=w1337) -> ("Input Command"=w1336:string, "Pump status"=w1332:string, "Valve position"=w1334:i32, "Absolute plunger position"=w1346:i32, "Serial port output"=w1341:string, "error out"=w1372:errorcluster)  [unwired: 2 in, 4 out]
        n376 = case shown="\"?\"" w1336 {
          tunnel: [w1382 w1388 w1393] -> w1353
          tunnel: w1352 -> [w1382 w1388 w1392]
          tunnel: w1351 -> [_ _ w1391]
          tunnel: w1346 -> [_ _ w1390]
          tunnel: w1333 -> [w1383 w1387 w1389]
          tunnel: [w1385 w1387 w1389] -> w1335
          tunnel: w1334 -> [w1384 _ _]
          frame "?6" {
            n377 = Build Array (concatenate)(w1383, w1384) -> (w1385:i32[])
            n378 = call "4155C Split array.vi"("Y1 data in"=w1385) -> ("Array of clusters"=w1386:cluster{"Y data in":dbl[], "X data in":dbl[]}[])  [unwired: 6 in, 1 out]
            n379 = local write "Valve position vs time"(w1386) -> ()
          }
          frame "Q", Default {
          }
          frame "?" {
            n380 = Build Array (concatenate)(w1392, w1390) -> (w1393:i32[])
            n381 = call "4155C Split array.vi"("X data in"=w1391, "Y1 data in"=w1393) -> ("Array of clusters"=w1394:cluster{"Y data in":dbl[], "X data in":dbl[]}[])  [unwired: 5 in, 1 out]
            n382 = local write "Absolute plunger position vs time"(w1394) -> ()
          }
        }
        n383 = Build Array (concatenate)(w1340, w1341) -> (w1366:string[])
      }
    }
    n384 = Build Array(w52, w103, w97) -> (w102:dbl[][])
    n385 = Build Array(w52, w53) -> (w61:i32[][])
    n386 = Concatenate Strings(w50, "Prefix (serial port output)", ".txt" ("Suffix")) -> (w79:string)
    n387 = Build Array(w54, "Id max /A" ("VAR2 Name"), "Id min /A" ("VAR2 Name")) -> (w108:string[])
    n388 = Build Array(w54, "Absolute plunger position" ("VAR2 Name")) -> (w64:string[])
    n389 = Array To Spreadsheet String(array=w80, 3:"" ("format string")) -> (spreadsheet string=w85:string)  [unwired: 1 in]
    n390 = Transpose 2D Array(2D array=w102) -> (transposed array=w101:dbl[][])
    n391 = Transpose 2D Array(2D array=w61) -> (transposed array=w51:i32[][])
    n392 = String To Path(string=w79) -> (path=w76:path)
    n393 = Concatenate Strings(w50, "Prefix (Idmax-Idmin)", "Suffix (Idmax-Idmin)") -> (w115:string)
    n394 = Array To Spreadsheet String(array=w64, 3:"" ("format string")) -> (spreadsheet string=w63:string)  [unwired: 1 in]
    n395 = Array To Spreadsheet String(array=w108, 3:"" ("format string")) -> (spreadsheet string=w107:string)  [unwired: 1 in]
    n396 = Array To Spreadsheet String(array=w101, 3:"%e" ("format string")) -> (spreadsheet string=w106:string)  [unwired: 1 in]
    n397 = Array To Spreadsheet String(array=w51, 3:"%e" ("format string")) -> (spreadsheet string=w60:string)  [unwired: 1 in]
    n398 = String To Path(string=w115) -> (path=w114:path)
    n399 = local write "Serial port data"(w85) -> ()
    n400 = Write to Text File(file (use dialog)=w76, text=w80, error in=w75) -> (refnum out=w81:refnum<file>, error out=w82:errorcluster)  [unwired: 1 in, 1 out]
    n401 = Build Array(w63, w60) -> (w66:string[])
    n402 = Build Array(w107, w106) -> (w105:string[])
    n403 = Close File(refnum=w81, error in=w82) -> (error out=w74:errorcluster)  [unwired: 1 out]
    n404 = Concatenate Strings(w50, "Prefix (plunger)", "Suffix (plunger)") -> (w58:string)
    n405 = String To Path(string=w58) -> (path=w55:path)
    n406 = Write to Text File(file (use dialog)=w114, text=w105, error in=w74) -> (refnum out=w116:refnum<file>, error out=w104:errorcluster)  [unwired: 1 in, 1 out]
    n407 = Write to Text File(file (use dialog)=w55, text=w66) -> (refnum out=w59:refnum<file>, error out=w68:errorcluster)  [unwired: 2 in, 1 out]
    n408 = Close File(refnum=w116, error in=w104) -> (error out=w99:errorcluster)  [unwired: 1 out]
    n409 = Close File(refnum=w59, error in=w68) -> ()  [unwired: 2 out]
  }
  "error out" <- w9
